vi "PIM Version.vi"() -> ()   [LabVIEW 2011]
uses:
  SI.LIB/OGAB Version.ctl
  server/database/Fields/Field Record.ctl
  server/database/Fields/Field DataTypes.ctl
  server/database/Fields/Field NextItem.ctl
panel:
  in  "Fields":T1[](array[typedef])=[{"ixField"=0, "iSequenceOrder"=0, "sxFieldId"="ALC", "sxSequenceId"="", "sDisplayName"="ALC", "sValue"="0", "sUnits"="", "nDataType"=enum."numeric", "nNextItem"=enum."Reset", "fSystem"=TRUE, "fSystemValue"=TRUE, "fRequired"=TRUE, "fSetAtTest"=TRUE, "fTestField"=TRUE, "fDeleted"=FALSE, "fIndexed"=FALSE, "fFreeList"=FALSE}, {"ixField"=0, "iSequenceOrder"=0, "sxFieldId"="Averaging", "sxSequenceId"="", "sDisplayName"="Averaging", "sValue"="None\tNone\tMinimum\tNormal\tHigh\tMaximum", "sUnits"="", "nDataType"=enum."list", "nNextItem"=enum."Reset", "fSystem"=TRUE, "fSystemValue"=TRUE, "fRequired"=TRUE, "fSetAtTest"=TRUE, "fTestField"=TRUE, "fDeleted"=FALSE, "fIndexed"=FALSE, "fFreeList"=FALSE}, {"ixField"=0, "iSequenceOrder"=0, "sxFieldId"="C1_Requested", "sxSequenceId"="", "sDisplayName"="C1 Requested", "sValue"="0", "sUnits"="dBm", "nDataType"=enum."numeric", "nNextItem"=enum."Reset", "fSystem"=TRUE, "fSystemValue"=TRUE, "fRequired"=TRUE, "fSetAtTest"=TRUE, "fTestField"=TRUE, "fDeleted"=FALSE, "fIndexed"=FALSE, "fFreeList"=FALSE}, {"ixField"=0, "iSequenceOrder"=0, "sxFieldId"="C2_Requested", "sxSequenceId"="", "sDisplayName"="C2 Requested", "sValue"="0", "sUnits"="dBm", "nDataType"=enum."numeric", "nNextItem"=enum."Reset", "fSystem"=TRUE, "fSystemValue"=TRUE, "fRequired"=TRUE, "fSetAtTest"=TRUE, "fTestField"=TRUE, "fDeleted"=FALSE, "fIndexed"=FALSE, "fFreeList"=FALSE}, {"ixField"=0, "iSequenceOrder"=0, "sxFieldId"="Calibration_Status", "sxSequenceId"="", "sDisplayName"="Calibration Status", "sValue"="0", "sUnits"="", "nDataType"=enum."numeric", "nNextItem"=enum."Reset", "fSystem"=TRUE, "fSystemValue"=TRUE, "fRequired"=TRUE, "fSetAtTest"=TRUE, "fTestField"=TRUE, "fDeleted"=FALSE, "fIndexed"=FALSE, "fFreeList"=FALSE}, {"ixField"=0, "iSequenceOrder"=0, "sxFieldId"="Cycles", "sxSequenceId"="", "sDisplayName"="Cycles", "sValue"="0", "sUnits"="", "nDataType"=enum."numeric", "nNextItem"=enum."Reset", "fSystem"=TRUE, "fSystemValue"=TRUE, "fRequired"=TRUE, "fSetAtTest"=TRUE, "fTestField"=TRUE, "fDeleted"=FALSE, "fIndexed"=FALSE, "fFreeList"=FALSE}, {"ixField"=0, "iSequenceOrder"=0, "sxFieldId"="DUT_Port", "sxSequenceId"="", "sDisplayName"="DUT Port", "sValue"="Port 1\tPort 1\tPort 2", "sUnits"="", "nDataType"=enum."list", "nNextItem"=enum."Reset", "fSystem"=TRUE, "fSystemValue"=TRUE, "fRequired"=TRUE, "fSetAtTest"=TRUE, "fTestField"=TRUE, "fDeleted"=FALSE, "fIndexed"=FALSE, "fFreeList"=FALSE}, {"ixField"=0, "iSequenceOrder"=0, "sxFieldId"="Display_Units_IM", "sxSequenceId"="", "sDisplayName"="Display Units IM", "sValue"="dBm\tdBm\tdBc", "sUnits"="", "nDataType"=enum."list", "nNextItem"=enum."Reset", "fSystem"=TRUE, "fSystemValue"=TRUE, "fRequired"=TRUE, "fSetAtTest"=TRUE, "fTestField"=TRUE, "fDeleted"=FALSE, "fIndexed"=FALSE, "fFreeList"=FALSE}, {"ixField"=0, "iSequenceOrder"=0, "sxFieldId"="Display_Units_Power", "sxSequenceId"="", "sDisplayName"="Display Units Power", "sValue"="dBm\tdBm\tWatts", "sUnits"="", "nDataType"=enum."list", "nNextItem"=enum."Reset", "fSystem"=TRUE, "fSystemValue"=TRUE, "fRequired"=TRUE, "fSetAtTest"=TRUE, "fTestField"=TRUE, "fDeleted"=FALSE, "fIndexed"=FALSE, "fFreeList"=FALSE}, {"ixField"=0, "iSequenceOrder"=0, "sxFieldId"="Display_Units_Samples", "sxSequenceId"="", "sDisplayName"="Display Units Samples", "sValue"="Sample(s)\tSample(s)\tSecond(s)\tSweep(s)", "sUnits"="", "nDataType"=enum."list", "nNextItem"=enum."Reset", "fSystem"=TRUE, "fSystemValue"=TRUE, "fRequired"=TRUE, "fSetAtTest"=TRUE, "fTestField"=TRUE, "fDeleted"=FALSE, "fIndexed"=FALSE, "fFreeList"=FALSE}, {"ixField"=0, "iSequenceOrder"=0, "sxFieldId"="IM11_Frequency_Average", "sxSequenceId"="", "sDisplayName"="IM11 Frequency Average", "sValue"="0", "sUnits"="MHz", "nDataType"=enum."numeric", "nNextItem"=enum."Reset", "fSystem"=TRUE, "fSystemValue"=TRUE, "fRequired"=TRUE, "fSetAtTest"=TRUE, "fTestField"=TRUE, "fDeleted"=FALSE, "fIndexed"=FALSE, "fFreeList"=FALSE}, {"ixField"=0, "iSequenceOrder"=0, "sxFieldId"="IM11_Frequency_Maximum", "sxSequenceId"="", "sDisplayName"="IM11 Frequency Maximum", "sValue"="0", "sUnits"="MHz", "nDataType"=enum."numeric", "nNextItem"=enum."Reset", "fSystem"=TRUE, "fSystemValue"=TRUE, "fRequired"=TRUE, "fSetAtTest"=TRUE, "fTestField"=TRUE, "fDeleted"=FALSE, "fIndexed"=FALSE, "fFreeList"=FALSE}, {"ixField"=0, "iSequenceOrder"=0, "sxFieldId"="IM11_Frequency_Minimum", "sxSequenceId"="", "sDisplayName"="IM11 Frequency Minimum", "sValue"="0", "sUnits"="MHz", "nDataType"=enum."numeric", "nNextItem"=enum."Reset", "fSystem"=TRUE, "fSystemValue"=TRUE, "fRequired"=TRUE, "fSetAtTest"=TRUE, "fTestField"=TRUE, "fDeleted"=FALSE, "fIndexed"=FALSE, "fFreeList"=FALSE}, {"ixField"=0, "iSequenceOrder"=0, "sxFieldId"="IM11_Frequency_Standard_Deviation", "sxSequenceId"="", "sDisplayName"="IM11 Frequency Standard Deviation", "sValue"="0", "sUnits"="MHz", "nDataType"=enum."numeric", "nNextItem"=enum."Reset", "fSystem"=TRUE, "fSystemValue"=TRUE, "fRequired"=TRUE, "fSetAtTest"=TRUE, "fTestField"=TRUE, "fDeleted"=FALSE, "fIndexed"=FALSE, "fFreeList"=FALSE}, {"ixField"=0, "iSequenceOrder"=0, "sxFieldId"="IM11_Power_1_Average", "sxSequenceId"="", "sDisplayName"="IM11 Power 1 Average", "sValue"="0", "sUnits"="dBm", "nDataType"=enum."numeric", "nNextItem"=enum."Reset", "fSystem"=TRUE, "fSystemValue"=TRUE, "fRequired"=TRUE, "fSetAtTest"=TRUE, "fTestField"=TRUE, "fDeleted"=FALSE, "fIndexed"=FALSE, "fFreeList"=FALSE}, {"ixField"=0, "iSequenceOrder"=0, "sxFieldId"="IM11_Power_1_Maximum", "sxSequenceId"="", "sDisplayName"="IM11 Power 1 Maximum", "sValue"="0", "sUnits"="dBm", "nDataType"=enum."numeric", "nNextItem"=enum."Reset", "fSystem"=TRUE, "fSystemValue"=TRUE, "fRequired"=TRUE, "fSetAtTest"=TRUE, "fTestField"=TRUE, "fDeleted"=FALSE, "fIndexed"=FALSE, "fFreeList"=FALSE}, {"ixField"=0, "iSequenceOrder"=0, "sxFieldId"="IM11_Power_1_Minimum", "sxSequenceId"="", "sDisplayName"="IM11 Power 1 Minimum", "sValue"="0", "sUnits"="dBm", "nDataType"=enum."numeric", "nNextItem"=enum."Reset", "fSystem"=TRUE, "fSystemValue"=TRUE, "fRequired"=TRUE, "fSetAtTest"=TRUE, "fTestField"=TRUE, "fDeleted"=FALSE, "fIndexed"=FALSE, "fFreeList"=FALSE}, {"ixField"=0, "iSequenceOrder"=0, "sxFieldId"="IM11_Power_1_Standard_Deviation", "sxSequenceId"="", "sDisplayName"="IM11 Power 1 Standard Deviation", "sValue"="0", "sUnits"="dBm", "nDataType"=enum."numeric", "nNextItem"=enum."Reset", "fSystem"=TRUE, "fSystemValue"=TRUE, "fRequired"=TRUE, "fSetAtTest"=TRUE, "fTestField"=TRUE, "fDeleted"=FALSE, "fIndexed"=FALSE, "fFreeList"=FALSE}, {"ixField"=0, "iSequenceOrder"=0, "sxFieldId"="IM11_Power_2_Average", "sxSequenceId"="", "sDisplayName"="IM11 Power 2 Average", "sValue"="0", "sUnits"="dBc", "nDataType"=enum."numeric", "nNextItem"=enum."Reset", "fSystem"=TRUE, "fSystemValue"=TRUE, "fRequired"=TRUE, "fSetAtTest"=TRUE, "fTestField"=TRUE, "fDeleted"=FALSE, "fIndexed"=FALSE, "fFreeList"=FALSE}, {"ixField"=0, "iSequenceOrder"=0, "sxFieldId"="IM11_Power_2_Maximum", "sxSequenceId"="", "sDisplayName"="IM11 Power 2 Maximum", "sValue"="0", "sUnits"="dBc", "nDataType"=enum."numeric", "nNextItem"=enum."Reset", "fSystem"=TRUE, "fSystemValue"=TRUE, "fRequired"=TRUE, "fSetAtTest"=TRUE, "fTestField"=TRUE, "fDeleted"=FALSE, "fIndexed"=FALSE, "fFreeList"=FALSE}, {"ixField"=0, "iSequenceOrder"=0, "sxFieldId"="IM11_Power_2_Minimum", "sxSequenceId"="", "sDisplayName"="IM11 Power 2 Minimum", "sValue"="0", "sUnits"="dBc", "nDataType"=enum."numeric", "nNextItem"=enum."Reset", "fSystem"=TRUE, "fSystemValue"=TRUE, "fRequired"=TRUE, "fSetAtTest"=TRUE, "fTestField"=TRUE, "fDeleted"=FALSE, "fIndexed"=FALSE, "fFreeList"=FALSE}, {"ixField"=0, "iSequenceOrder"=0, "sxFieldId"="IM11_Power_2_Standard_Deviation", "sxSequenceId"="", "sDisplayName"="IM11 Power 2 Standard Deviation", "sValue"="0", "sUnits"="dBc", "nDataType"=enum."numeric", "nNextItem"=enum."Reset", "fSystem"=TRUE, "fSystemValue"=TRUE, "fRequired"=TRUE, "fSetAtTest"=TRUE, "fTestField"=TRUE, "fDeleted"=FALSE, "fIndexed"=FALSE, "fFreeList"=FALSE}, {"ixField"=0, "iSequenceOrder"=0, "sxFieldId"="IM13_Frequency_Average", "sxSequenceId"="", "sDisplayName"="IM13 Frequency Average", "sValue"="0", "sUnits"="MHz", "nDataType"=enum."numeric", "nNextItem"=enum."Reset", "fSystem"=TRUE, "fSystemValue"=TRUE, "fRequired"=TRUE, "fSetAtTest"=TRUE, "fTestField"=TRUE, "fDeleted"=FALSE, "fIndexed"=FALSE, "fFreeList"=FALSE}, {"ixField"=0, "iSequenceOrder"=0, "sxFieldId"="IM13_Frequency_Maximum", "sxSequenceId"="", "sDisplayName"="IM13 Frequency Maximum", "sValue"="0", "sUnits"="MHz", "nDataType"=enum."numeric", "nNextItem"=enum."Reset", "fSystem"=TRUE, "fSystemValue"=TRUE, "fRequired"=TRUE, "fSetAtTest"=TRUE, "fTestField"=TRUE, "fDeleted"=FALSE, "fIndexed"=FALSE, "fFreeList"=FALSE}, {"ixField"=0, "iSequenceOrder"=0, "sxFieldId"="IM13_Frequency_Minimum", "sxSequenceId"="", "sDisplayName"="IM13 Frequency Minimum", "sValue"="0", "sUnits"="MHz", "nDataType"=enum."numeric", "nNextItem"=enum."Reset", "fSystem"=TRUE, "fSystemValue"=TRUE, "fRequired"=TRUE, "fSetAtTest"=TRUE, "fTestField"=TRUE, "fDeleted"=FALSE, "fIndexed"=FALSE, "fFreeList"=FALSE}, {"ixField"=0, "iSequenceOrder"=0, "sxFieldId"="IM13_Frequency_Standard_Deviation", "sxSequenceId"="", "sDisplayName"="IM13 Frequency Standard Deviation", "sValue"="0", "sUnits"="MHz", "nDataType"=enum."numeric", "nNextItem"=enum."Reset", "fSystem"=TRUE, "fSystemValue"=TRUE, "fRequired"=TRUE, "fSetAtTest"=TRUE, "fTestField"=TRUE, "fDeleted"=FALSE, "fIndexed"=FALSE, "fFreeList"=FALSE}, {"ixField"=0, "iSequenceOrder"=0, "sxFieldId"="IM13_Power_1_Average", "sxSequenceId"="", "sDisplayName"="IM13 Power 1 Average", "sValue"="0", "sUnits"="dBm", "nDataType"=enum."numeric", "nNextItem"=enum."Reset", "fSystem"=TRUE, "fSystemValue"=TRUE, "fRequired"=TRUE, "fSetAtTest"=TRUE, "fTestField"=TRUE, "fDeleted"=FALSE, "fIndexed"=FALSE, "fFreeList"=FALSE}, {"ixField"=0, "iSequenceOrder"=0, "sxFieldId"="IM13_Power_1_Maximum", "sxSequenceId"="", "sDisplayName"="IM13 Power 1 Maximum", "sValue"="0", "sUnits"="dBm", "nDataType"=enum."numeric", "nNextItem"=enum."Reset", "fSystem"=TRUE, "fSystemValue"=TRUE, "fRequired"=TRUE, "fSetAtTest"=TRUE, "fTestField"=TRUE, "fDeleted"=FALSE, "fIndexed"=FALSE, "fFreeList"=FALSE}, {"ixField"=0, "iSequenceOrder"=0, "sxFieldId"="IM13_Power_1_Minimum", "sxSequenceId"="", "sDisplayName"="IM13 Power 1 Minimum", "sValue"="0", "sUnits"="dBm", "nDataType"=enum."numeric", "nNextItem"=enum."Reset", "fSystem"=TRUE, "fSystemValue"=TRUE, "fRequired"=TRUE, "fSetAtTest"=TRUE, "fTestField"=TRUE, "fDeleted"=FALSE, "fIndexed"=FALSE, "fFreeList"=FALSE}, {"ixField"=0, "iSequenceOrder"=0, "sxFieldId"="IM13_Power_1_Standard_Deviation", "sxSequenceId"="", "sDisplayName"="IM13 Power 1 Standard Deviation", "sValue"="0", "sUnits"="dBm", "nDataType"=enum."numeric", "nNextItem"=enum."Reset", "fSystem"=TRUE, "fSystemValue"=TRUE, "fRequired"=TRUE, "fSetAtTest"=TRUE, "fTestField"=TRUE, "fDeleted"=FALSE, "fIndexed"=FALSE, "fFreeList"=FALSE}, {"ixField"=0, "iSequenceOrder"=0, "sxFieldId"="IM13_Power_2_Average", "sxSequenceId"="", "sDisplayName"="IM13 Power 2 Average", "sValue"="0", "sUnits"="dBc", "nDataType"=enum."numeric", "nNextItem"=enum."Reset", "fSystem"=TRUE, "fSystemValue"=TRUE, "fRequired"=TRUE, "fSetAtTest"=TRUE, "fTestField"=TRUE, "fDeleted"=FALSE, "fIndexed"=FALSE, "fFreeList"=FALSE}, {"ixField"=0, "iSequenceOrder"=0, "sxFieldId"="IM13_Power_2_Maximum", "sxSequenceId"="", "sDisplayName"="IM13 Power 2 Maximum", "sValue"="0", "sUnits"="dBc", "nDataType"=enum."numeric", "nNextItem"=enum."Reset", "fSystem"=TRUE, "fSystemValue"=TRUE, "fRequired"=TRUE, "fSetAtTest"=TRUE, "fTestField"=TRUE, "fDeleted"=FALSE, "fIndexed"=FALSE, "fFreeList"=FALSE}, {"ixField"=0, "iSequenceOrder"=0, "sxFieldId"="IM13_Power_2_Minimum", "sxSequenceId"="", "sDisplayName"="IM13 Power 2 Minimum", "sValue"="0", "sUnits"="dBc", "nDataType"=enum."numeric", "nNextItem"=enum."Reset", "fSystem"=TRUE, "fSystemValue"=TRUE, "fRequired"=TRUE, "fSetAtTest"=TRUE, "fTestField"=TRUE, "fDeleted"=FALSE, "fIndexed"=FALSE, "fFreeList"=FALSE}, {"ixField"=0, "iSequenceOrder"=0, "sxFieldId"="IM13_Power_2_Standard_Deviation", "sxSequenceId"="", "sDisplayName"="IM13 Power 2 Standard Deviation", "sValue"="0", "sUnits"="dBc", "nDataType"=enum."numeric", "nNextItem"=enum."Reset", "fSystem"=TRUE, "fSystemValue"=TRUE, "fRequired"=TRUE, "fSetAtTest"=TRUE, "fTestField"=TRUE, "fDeleted"=FALSE, "fIndexed"=FALSE, "fFreeList"=FALSE}, {"ixField"=0, "iSequenceOrder"=0, "sxFieldId"="IM15_Frequency_Average", "sxSequenceId"="", "sDisplayName"="IM15 Frequency Average", "sValue"="0", "sUnits"="MHz", "nDataType"=enum."numeric", "nNextItem"=enum."Reset", "fSystem"=TRUE, "fSystemValue"=TRUE, "fRequired"=TRUE, "fSetAtTest"=TRUE, "fTestField"=TRUE, "fDeleted"=FALSE, "fIndexed"=FALSE, "fFreeList"=FALSE}, {"ixField"=0, "iSequenceOrder"=0, "sxFieldId"="IM15_Frequency_Maximum", "sxSequenceId"="", "sDisplayName"="IM15 Frequency Maximum", "sValue"="0", "sUnits"="MHz", "nDataType"=enum."numeric", "nNextItem"=enum."Reset", "fSystem"=TRUE, "fSystemValue"=TRUE, "fRequired"=TRUE, "fSetAtTest"=TRUE, "fTestField"=TRUE, "fDeleted"=FALSE, "fIndexed"=FALSE, "fFreeList"=FALSE}, {"ixField"=0, "iSequenceOrder"=0, "sxFieldId"="IM15_Frequency_Minimum", "sxSequenceId"="", "sDisplayName"="IM15 Frequency Minimum", "sValue"="0", "sUnits"="MHz", "nDataType"=enum."numeric", "nNextItem"=enum."Reset", "fSystem"=TRUE, "fSystemValue"=TRUE, "fRequired"=TRUE, "fSetAtTest"=TRUE, "fTestField"=TRUE, "fDeleted"=FALSE, "fIndexed"=FALSE, "fFreeList"=FALSE}, {"ixField"=0, "iSequenceOrder"=0, "sxFieldId"="IM15_Frequency_Standard_Deviation", "sxSequenceId"="", "sDisplayName"="IM15 Frequency Standard Deviation", "sValue"="0", "sUnits"="MHz", "nDataType"=enum."numeric", "nNextItem"=enum."Reset", "fSystem"=TRUE, "fSystemValue"=TRUE, "fRequired"=TRUE, "fSetAtTest"=TRUE, "fTestField"=TRUE, "fDeleted"=FALSE, "fIndexed"=FALSE, "fFreeList"=FALSE}, {"ixField"=0, "iSequenceOrder"=0, "sxFieldId"="IM15_Power_1_Average", "sxSequenceId"="", "sDisplayName"="IM15 Power 1 Average", "sValue"="0", "sUnits"="dBm", "nDataType"=enum."numeric", "nNextItem"=enum."Reset", "fSystem"=TRUE, "fSystemValue"=TRUE, "fRequired"=TRUE, "fSetAtTest"=TRUE, "fTestField"=TRUE, "fDeleted"=FALSE, "fIndexed"=FALSE, "fFreeList"=FALSE}, {"ixField"=0, "iSequenceOrder"=0, "sxFieldId"="IM15_Power_1_Maximum", "sxSequenceId"="", "sDisplayName"="IM15 Power 1 Maximum", "sValue"="0", "sUnits"="dBm", "nDataType"=enum."numeric", "nNextItem"=enum."Reset", "fSystem"=TRUE, "fSystemValue"=TRUE, "fRequired"=TRUE, "fSetAtTest"=TRUE, "fTestField"=TRUE, "fDeleted"=FALSE, "fIndexed"=FALSE, "fFreeList"=FALSE}, {"ixField"=0, "iSequenceOrder"=0, "sxFieldId"="IM15_Power_1_Minimum", "sxSequenceId"="", "sDisplayName"="IM15 Power 1 Minimum", "sValue"="0", "sUnits"="dBm", "nDataType"=enum."numeric", "nNextItem"=enum."Reset", "fSystem"=TRUE, "fSystemValue"=TRUE, "fRequired"=TRUE, "fSetAtTest"=TRUE, "fTestField"=TRUE, "fDeleted"=FALSE, "fIndexed"=FALSE, "fFreeList"=FALSE}, {"ixField"=0, "iSequenceOrder"=0, "sxFieldId"="IM15_Power_1_Standard_Deviation", "sxSequenceId"="", "sDisplayName"="IM15 Power 1 Standard Deviation", "sValue"="0", "sUnits"="dBm", "nDataType"=enum."numeric", "nNextItem"=enum."Reset", "fSystem"=TRUE, "fSystemValue"=TRUE, "fRequired"=TRUE, "fSetAtTest"=TRUE, "fTestField"=TRUE, "fDeleted"=FALSE, "fIndexed"=FALSE, "fFreeList"=FALSE}, {"ixField"=0, "iSequenceOrder"=0, "sxFieldId"="IM15_Power_2_Average", "sxSequenceId"="", "sDisplayName"="IM15 Power 2 Average", "sValue"="0", "sUnits"="dBc", "nDataType"=enum."numeric", "nNextItem"=enum."Reset", "fSystem"=TRUE, "fSystemValue"=TRUE, "fRequired"=TRUE, "fSetAtTest"=TRUE, "fTestField"=TRUE, "fDeleted"=FALSE, "fIndexed"=FALSE, "fFreeList"=FALSE}, {"ixField"=0, "iSequenceOrder"=0, "sxFieldId"="IM15_Power_2_Maximum", "sxSequenceId"="", "sDisplayName"="IM15 Power 2 Maximum", "sValue"="0", "sUnits"="dBc", "nDataType"=enum."numeric", "nNextItem"=enum."Reset", "fSystem"=TRUE, "fSystemValue"=TRUE, "fRequired"=TRUE, "fSetAtTest"=TRUE, "fTestField"=TRUE, "fDeleted"=FALSE, "fIndexed"=FALSE, "fFreeList"=FALSE}, {"ixField"=0, "iSequenceOrder"=0, "sxFieldId"="IM15_Power_2_Minimum", "sxSequenceId"="", "sDisplayName"="IM15 Power 2 Minimum", "sValue"="0", "sUnits"="dBc", "nDataType"=enum."numeric", "nNextItem"=enum."Reset", "fSystem"=TRUE, "fSystemValue"=TRUE, "fRequired"=TRUE, "fSetAtTest"=TRUE, "fTestField"=TRUE, "fDeleted"=FALSE, "fIndexed"=FALSE, "fFreeList"=FALSE}, {"ixField"=0, "iSequenceOrder"=0, "sxFieldId"="IM15_Power_2_Standard_Deviation", "sxSequenceId"="", "sDisplayName"="IM15 Power 2 Standard Deviation", "sValue"="0", "sUnits"="dBc", "nDataType"=enum."numeric", "nNextItem"=enum."Reset", "fSystem"=TRUE, "fSystemValue"=TRUE, "fRequired"=TRUE, "fSetAtTest"=TRUE, "fTestField"=TRUE, "fDeleted"=FALSE, "fIndexed"=FALSE, "fFreeList"=FALSE}, {"ixField"=0, "iSequenceOrder"=0, "sxFieldId"="IM17_Frequency_Average", "sxSequenceId"="", "sDisplayName"="IM17 Frequency Average", "sValue"="0", "sUnits"="MHz", "nDataType"=enum."numeric", "nNextItem"=enum."Reset", "fSystem"=TRUE, "fSystemValue"=TRUE, "fRequired"=TRUE, "fSetAtTest"=TRUE, "fTestField"=TRUE, "fDeleted"=FALSE, "fIndexed"=FALSE, "fFreeList"=FALSE}, {"ixField"=0, "iSequenceOrder"=0, "sxFieldId"="IM17_Frequency_Maximum", "sxSequenceId"="", "sDisplayName"="IM17 Frequency Maximum", "sValue"="0", "sUnits"="MHz", "nDataType"=enum."numeric", "nNextItem"=enum."Reset", "fSystem"=TRUE, "fSystemValue"=TRUE, "fRequired"=TRUE, "fSetAtTest"=TRUE, "fTestField"=TRUE, "fDeleted"=FALSE, "fIndexed"=FALSE, "fFreeList"=FALSE}, {"ixField"=0, "iSequenceOrder"=0, "sxFieldId"="IM17_Frequency_Minimum", "sxSequenceId"="", "sDisplayName"="IM17 Frequency Minimum", "sValue"="0", "sUnits"="MHz", "nDataType"=enum."numeric", "nNextItem"=enum."Reset", "fSystem"=TRUE, "fSystemValue"=TRUE, "fRequired"=TRUE, "fSetAtTest"=TRUE, "fTestField"=TRUE, "fDeleted"=FALSE, "fIndexed"=FALSE, "fFreeList"=FALSE}, {"ixField"=0, "iSequenceOrder"=0, "sxFieldId"="IM17_Frequency_Standard_Deviation", "sxSequenceId"="", "sDisplayName"="IM17 Frequency Standard Deviation", "sValue"="0", "sUnits"="MHz", "nDataType"=enum."numeric", "nNextItem"=enum."Reset", "fSystem"=TRUE, "fSystemValue"=TRUE, "fRequired"=TRUE, "fSetAtTest"=TRUE, "fTestField"=TRUE, "fDeleted"=FALSE, "fIndexed"=FALSE, "fFreeList"=FALSE}, {"ixField"=0, "iSequenceOrder"=0, "sxFieldId"="IM17_Power_1_Average", "sxSequenceId"="", "sDisplayName"="IM17 Power 1 Average", "sValue"="0", "sUnits"="dBm", "nDataType"=enum."numeric", "nNextItem"=enum."Reset", "fSystem"=TRUE, "fSystemValue"=TRUE, "fRequired"=TRUE, "fSetAtTest"=TRUE, "fTestField"=TRUE, "fDeleted"=FALSE, "fIndexed"=FALSE, "fFreeList"=FALSE}, {"ixField"=0, "iSequenceOrder"=0, "sxFieldId"="IM17_Power_1_Maximum", "sxSequenceId"="", "sDisplayName"="IM17 Power 1 Maximum", "sValue"="0", "sUnits"="dBm", "nDataType"=enum."numeric", "nNextItem"=enum."Reset", "fSystem"=TRUE, "fSystemValue"=TRUE, "fRequired"=TRUE, "fSetAtTest"=TRUE, "fTestField"=TRUE, "fDeleted"=FALSE, "fIndexed"=FALSE, "fFreeList"=FALSE}, {"ixField"=0, "iSequenceOrder"=0, "sxFieldId"="IM17_Power_1_Minimum", "sxSequenceId"="", "sDisplayName"="IM17 Power 1 Minimum", "sValue"="0", "sUnits"="dBm", "nDataType"=enum."numeric", "nNextItem"=enum."Reset", "fSystem"=TRUE, "fSystemValue"=TRUE, "fRequired"=TRUE, "fSetAtTest"=TRUE, "fTestField"=TRUE, "fDeleted"=FALSE, "fIndexed"=FALSE, "fFreeList"=FALSE}, {"ixField"=0, "iSequenceOrder"=0, "sxFieldId"="IM17_Power_1_Standard_Deviation", "sxSequenceId"="", "sDisplayName"="IM17 Power 1 Standard Deviation", "sValue"="0", "sUnits"="dBm", "nDataType"=enum."numeric", "nNextItem"=enum."Reset", "fSystem"=TRUE, "fSystemValue"=TRUE, "fRequired"=TRUE, "fSetAtTest"=TRUE, "fTestField"=TRUE, "fDeleted"=FALSE, "fIndexed"=FALSE, "fFreeList"=FALSE}, {"ixField"=0, "iSequenceOrder"=0, "sxFieldId"="IM17_Power_2_Average", "sxSequenceId"="", "sDisplayName"="IM17 Power 2 Average", "sValue"="0", "sUnits"="dBc", "nDataType"=enum."numeric", "nNextItem"=enum."Reset", "fSystem"=TRUE, "fSystemValue"=TRUE, "fRequired"=TRUE, "fSetAtTest"=TRUE, "fTestField"=TRUE, "fDeleted"=FALSE, "fIndexed"=FALSE, "fFreeList"=FALSE}, {"ixField"=0, "iSequenceOrder"=0, "sxFieldId"="IM17_Power_2_Maximum", "sxSequenceId"="", "sDisplayName"="IM17 Power 2 Maximum", "sValue"="0", "sUnits"="dBc", "nDataType"=enum."numeric", "nNextItem"=enum."Reset", "fSystem"=TRUE, "fSystemValue"=TRUE, "fRequired"=TRUE, "fSetAtTest"=TRUE, "fTestField"=TRUE, "fDeleted"=FALSE, "fIndexed"=FALSE, "fFreeList"=FALSE}, {"ixField"=0, "iSequenceOrder"=0, "sxFieldId"="IM17_Power_2_Minimum", "sxSequenceId"="", "sDisplayName"="IM17 Power 2 Minimum", "sValue"="0", "sUnits"="dBc", "nDataType"=enum."numeric", "nNextItem"=enum."Reset", "fSystem"=TRUE, "fSystemValue"=TRUE, "fRequired"=TRUE, "fSetAtTest"=TRUE, "fTestField"=TRUE, "fDeleted"=FALSE, "fIndexed"=FALSE, "fFreeList"=FALSE}, {"ixField"=0, "iSequenceOrder"=0, "sxFieldId"="IM17_Power_2_Standard_Deviation", "sxSequenceId"="", "sDisplayName"="IM17 Power 2 Standard Deviation", "sValue"="0", "sUnits"="dBc", "nDataType"=enum."numeric", "nNextItem"=enum."Reset", "fSystem"=TRUE, "fSystemValue"=TRUE, "fRequired"=TRUE, "fSetAtTest"=TRUE, "fTestField"=TRUE, "fDeleted"=FALSE, "fIndexed"=FALSE, "fFreeList"=FALSE}, {"ixField"=0, "iSequenceOrder"=0, "sxFieldId"="IM19_Frequency_Average", "sxSequenceId"="", "sDisplayName"="IM19 Frequency Average", "sValue"="0", "sUnits"="MHz", "nDataType"=enum."numeric", "nNextItem"=enum."Reset", "fSystem"=TRUE, "fSystemValue"=TRUE, "fRequired"=TRUE, "fSetAtTest"=TRUE, "fTestField"=TRUE, "fDeleted"=FALSE, "fIndexed"=FALSE, "fFreeList"=FALSE}, {"ixField"=0, "iSequenceOrder"=0, "sxFieldId"="IM19_Frequency_Maximum", "sxSequenceId"="", "sDisplayName"="IM19 Frequency Maximum", "sValue"="0", "sUnits"="MHz", "nDataType"=enum."numeric", "nNextItem"=enum."Reset", "fSystem"=TRUE, "fSystemValue"=TRUE, "fRequired"=TRUE, "fSetAtTest"=TRUE, "fTestField"=TRUE, "fDeleted"=FALSE, "fIndexed"=FALSE, "fFreeList"=FALSE}, {"ixField"=0, "iSequenceOrder"=0, "sxFieldId"="IM19_Frequency_Minimum", "sxSequenceId"="", "sDisplayName"="IM19 Frequency Minimum", "sValue"="0", "sUnits"="MHz", "nDataType"=enum."numeric", "nNextItem"=enum."Reset", "fSystem"=TRUE, "fSystemValue"=TRUE, "fRequired"=TRUE, "fSetAtTest"=TRUE, "fTestField"=TRUE, "fDeleted"=FALSE, "fIndexed"=FALSE, "fFreeList"=FALSE}, {"ixField"=0, "iSequenceOrder"=0, "sxFieldId"="IM19_Frequency_Standard_Deviation", "sxSequenceId"="", "sDisplayName"="IM19 Frequency Standard Deviation", "sValue"="0", "sUnits"="MHz", "nDataType"=enum."numeric", "nNextItem"=enum."Reset", "fSystem"=TRUE, "fSystemValue"=TRUE, "fRequired"=TRUE, "fSetAtTest"=TRUE, "fTestField"=TRUE, "fDeleted"=FALSE, "fIndexed"=FALSE, "fFreeList"=FALSE}, {"ixField"=0, "iSequenceOrder"=0, "sxFieldId"="IM19_Power_1_Average", "sxSequenceId"="", "sDisplayName"="IM19 Power 1 Average", "sValue"="0", "sUnits"="dBm", "nDataType"=enum."numeric", "nNextItem"=enum."Reset", "fSystem"=TRUE, "fSystemValue"=TRUE, "fRequired"=TRUE, "fSetAtTest"=TRUE, "fTestField"=TRUE, "fDeleted"=FALSE, "fIndexed"=FALSE, "fFreeList"=FALSE}, {"ixField"=0, "iSequenceOrder"=0, "sxFieldId"="IM19_Power_1_Maximum", "sxSequenceId"="", "sDisplayName"="IM19 Power 1 Maximum", "sValue"="0", "sUnits"="dBm", "nDataType"=enum."numeric", "nNextItem"=enum."Reset", "fSystem"=TRUE, "fSystemValue"=TRUE, "fRequired"=TRUE, "fSetAtTest"=TRUE, "fTestField"=TRUE, "fDeleted"=FALSE, "fIndexed"=FALSE, "fFreeList"=FALSE}, {"ixField"=0, "iSequenceOrder"=0, "sxFieldId"="IM19_Power_1_Minimum", "sxSequenceId"="", "sDisplayName"="IM19 Power 1 Minimum", "sValue"="0", "sUnits"="dBm", "nDataType"=enum."numeric", "nNextItem"=enum."Reset", "fSystem"=TRUE, "fSystemValue"=TRUE, "fRequired"=TRUE, "fSetAtTest"=TRUE, "fTestField"=TRUE, "fDeleted"=FALSE, "fIndexed"=FALSE, "fFreeList"=FALSE}, {"ixField"=0, "iSequenceOrder"=0, "sxFieldId"="IM19_Power_1_Standard_Deviation", "sxSequenceId"="", "sDisplayName"="IM19 Power 1 Standard Deviation", "sValue"="0", "sUnits"="dBm", "nDataType"=enum."numeric", "nNextItem"=enum."Reset", "fSystem"=TRUE, "fSystemValue"=TRUE, "fRequired"=TRUE, "fSetAtTest"=TRUE, "fTestField"=TRUE, "fDeleted"=FALSE, "fIndexed"=FALSE, "fFreeList"=FALSE}, {"ixField"=0, "iSequenceOrder"=0, "sxFieldId"="IM19_Power_2_Average", "sxSequenceId"="", "sDisplayName"="IM19 Power 2 Average", "sValue"="0", "sUnits"="dBc", "nDataType"=enum."numeric", "nNextItem"=enum."Reset", "fSystem"=TRUE, "fSystemValue"=TRUE, "fRequired"=TRUE, "fSetAtTest"=TRUE, "fTestField"=TRUE, "fDeleted"=FALSE, "fIndexed"=FALSE, "fFreeList"=FALSE}, {"ixField"=0, "iSequenceOrder"=0, "sxFieldId"="IM19_Power_2_Maximum", "sxSequenceId"="", "sDisplayName"="IM19 Power 2 Maximum", "sValue"="0", "sUnits"="dBc", "nDataType"=enum."numeric", "nNextItem"=enum."Reset", "fSystem"=TRUE, "fSystemValue"=TRUE, "fRequired"=TRUE, "fSetAtTest"=TRUE, "fTestField"=TRUE, "fDeleted"=FALSE, "fIndexed"=FALSE, "fFreeList"=FALSE}, {"ixField"=0, "iSequenceOrder"=0, "sxFieldId"="IM19_Power_2_Minimum", "sxSequenceId"="", "sDisplayName"="IM19 Power 2 Minimum", "sValue"="0", "sUnits"="dBc", "nDataType"=enum."numeric", "nNextItem"=enum."Reset", "fSystem"=TRUE, "fSystemValue"=TRUE, "fRequired"=TRUE, "fSetAtTest"=TRUE, "fTestField"=TRUE, "fDeleted"=FALSE, "fIndexed"=FALSE, "fFreeList"=FALSE}, {"ixField"=0, "iSequenceOrder"=0, "sxFieldId"="IM19_Power_2_Standard_Deviation", "sxSequenceId"="", "sDisplayName"="IM19 Power 2 Standard Deviation", "sValue"="0", "sUnits"="dBc", "nDataType"=enum."numeric", "nNextItem"=enum."Reset", "fSystem"=TRUE, "fSystemValue"=TRUE, "fRequired"=TRUE, "fSetAtTest"=TRUE, "fTestField"=TRUE, "fDeleted"=FALSE, "fIndexed"=FALSE, "fFreeList"=FALSE}, {"ixField"=0, "iSequenceOrder"=0, "sxFieldId"="IM21_Frequency_Average", "sxSequenceId"="", "sDisplayName"="IM21 Frequency Average", "sValue"="0", "sUnits"="MHz", "nDataType"=enum."numeric", "nNextItem"=enum."Reset", "fSystem"=TRUE, "fSystemValue"=TRUE, "fRequired"=TRUE, "fSetAtTest"=TRUE, "fTestField"=TRUE, "fDeleted"=FALSE, "fIndexed"=FALSE, "fFreeList"=FALSE}, {"ixField"=0, "iSequenceOrder"=0, "sxFieldId"="IM21_Frequency_Maximum", "sxSequenceId"="", "sDisplayName"="IM21 Frequency Maximum", "sValue"="0", "sUnits"="MHz", "nDataType"=enum."numeric", "nNextItem"=enum."Reset", "fSystem"=TRUE, "fSystemValue"=TRUE, "fRequired"=TRUE, "fSetAtTest"=TRUE, "fTestField"=TRUE, "fDeleted"=FALSE, "fIndexed"=FALSE, "fFreeList"=FALSE}, {"ixField"=0, "iSequenceOrder"=0, "sxFieldId"="IM21_Frequency_Minimum", "sxSequenceId"="", "sDisplayName"="IM21 Frequency Minimum", "sValue"="0", "sUnits"="MHz", "nDataType"=enum."numeric", "nNextItem"=enum."Reset", "fSystem"=TRUE, "fSystemValue"=TRUE, "fRequired"=TRUE, "fSetAtTest"=TRUE, "fTestField"=TRUE, "fDeleted"=FALSE, "fIndexed"=FALSE, "fFreeList"=FALSE}, {"ixField"=0, "iSequenceOrder"=0, "sxFieldId"="IM21_Frequency_Standard_Deviation", "sxSequenceId"="", "sDisplayName"="IM21 Frequency Standard Deviation", "sValue"="0", "sUnits"="MHz", "nDataType"=enum."numeric", "nNextItem"=enum."Reset", "fSystem"=TRUE, "fSystemValue"=TRUE, "fRequired"=TRUE, "fSetAtTest"=TRUE, "fTestField"=TRUE, "fDeleted"=FALSE, "fIndexed"=FALSE, "fFreeList"=FALSE}, {"ixField"=0, "iSequenceOrder"=0, "sxFieldId"="IM21_Power_1_Average", "sxSequenceId"="", "sDisplayName"="IM21 Power 1 Average", "sValue"="0", "sUnits"="dBm", "nDataType"=enum."numeric", "nNextItem"=enum."Reset", "fSystem"=TRUE, "fSystemValue"=TRUE, "fRequired"=TRUE, "fSetAtTest"=TRUE, "fTestField"=TRUE, "fDeleted"=FALSE, "fIndexed"=FALSE, "fFreeList"=FALSE}, {"ixField"=0, "iSequenceOrder"=0, "sxFieldId"="IM21_Power_1_Maximum", "sxSequenceId"="", "sDisplayName"="IM21 Power 1 Maximum", "sValue"="0", "sUnits"="dBm", "nDataType"=enum."numeric", "nNextItem"=enum."Reset", "fSystem"=TRUE, "fSystemValue"=TRUE, "fRequired"=TRUE, "fSetAtTest"=TRUE, "fTestField"=TRUE, "fDeleted"=FALSE, "fIndexed"=FALSE, "fFreeList"=FALSE}, {"ixField"=0, "iSequenceOrder"=0, "sxFieldId"="IM21_Power_1_Minimum", "sxSequenceId"="", "sDisplayName"="IM21 Power 1 Minimum", "sValue"="0", "sUnits"="dBm", "nDataType"=enum."numeric", "nNextItem"=enum."Reset", "fSystem"=TRUE, "fSystemValue"=TRUE, "fRequired"=TRUE, "fSetAtTest"=TRUE, "fTestField"=TRUE, "fDeleted"=FALSE, "fIndexed"=FALSE, "fFreeList"=FALSE}, {"ixField"=0, "iSequenceOrder"=0, "sxFieldId"="IM21_Power_1_Standard_Deviation", "sxSequenceId"="", "sDisplayName"="IM21 Power 1 Standard Deviation", "sValue"="0", "sUnits"="dBm", "nDataType"=enum."numeric", "nNextItem"=enum."Reset", "fSystem"=TRUE, "fSystemValue"=TRUE, "fRequired"=TRUE, "fSetAtTest"=TRUE, "fTestField"=TRUE, "fDeleted"=FALSE, "fIndexed"=FALSE, "fFreeList"=FALSE}, {"ixField"=0, "iSequenceOrder"=0, "sxFieldId"="IM21_Power_2_Average", "sxSequenceId"="", "sDisplayName"="IM21 Power 2 Average", "sValue"="0", "sUnits"="dBc", "nDataType"=enum."numeric", "nNextItem"=enum."Reset", "fSystem"=TRUE, "fSystemValue"=TRUE, "fRequired"=TRUE, "fSetAtTest"=TRUE, "fTestField"=TRUE, "fDeleted"=FALSE, "fIndexed"=FALSE, "fFreeList"=FALSE}, {"ixField"=0, "iSequenceOrder"=0, "sxFieldId"="IM21_Power_2_Maximum", "sxSequenceId"="", "sDisplayName"="IM21 Power 2 Maximum", "sValue"="0", "sUnits"="dBc", "nDataType"=enum."numeric", "nNextItem"=enum."Reset", "fSystem"=TRUE, "fSystemValue"=TRUE, "fRequired"=TRUE, "fSetAtTest"=TRUE, "fTestField"=TRUE, "fDeleted"=FALSE, "fIndexed"=FALSE, "fFreeList"=FALSE}, {"ixField"=0, "iSequenceOrder"=0, "sxFieldId"="IM21_Power_2_Minimum", "sxSequenceId"="", "sDisplayName"="IM21 Power 2 Minimum", "sValue"="0", "sUnits"="dBc", "nDataType"=enum."numeric", "nNextItem"=enum."Reset", "fSystem"=TRUE, "fSystemValue"=TRUE, "fRequired"=TRUE, "fSetAtTest"=TRUE, "fTestField"=TRUE, "fDeleted"=FALSE, "fIndexed"=FALSE, "fFreeList"=FALSE}, {"ixField"=0, "iSequenceOrder"=0, "sxFieldId"="IM21_Power_2_Standard_Deviation", "sxSequenceId"="", "sDisplayName"="IM21 Power 2 Standard Deviation", "sValue"="0", "sUnits"="dBc", "nDataType"=enum."numeric", "nNextItem"=enum."Reset", "fSystem"=TRUE, "fSystemValue"=TRUE, "fRequired"=TRUE, "fSetAtTest"=TRUE, "fTestField"=TRUE, "fDeleted"=FALSE, "fIndexed"=FALSE, "fFreeList"=FALSE}, {"ixField"=0, "iSequenceOrder"=0, "sxFieldId"="IM23_Frequency_Average", "sxSequenceId"="", "sDisplayName"="IM23 Frequency Average", "sValue"="0", "sUnits"="MHz", "nDataType"=enum."numeric", "nNextItem"=enum."Reset", "fSystem"=TRUE, "fSystemValue"=TRUE, "fRequired"=TRUE, "fSetAtTest"=TRUE, "fTestField"=TRUE, "fDeleted"=FALSE, "fIndexed"=FALSE, "fFreeList"=FALSE}, {"ixField"=0, "iSequenceOrder"=0, "sxFieldId"="IM23_Frequency_Maximum", "sxSequenceId"="", "sDisplayName"="IM23 Frequency Maximum", "sValue"="0", "sUnits"="MHz", "nDataType"=enum."numeric", "nNextItem"=enum."Reset", "fSystem"=TRUE, "fSystemValue"=TRUE, "fRequired"=TRUE, "fSetAtTest"=TRUE, "fTestField"=TRUE, "fDeleted"=FALSE, "fIndexed"=FALSE, "fFreeList"=FALSE}, {"ixField"=0, "iSequenceOrder"=0, "sxFieldId"="IM23_Frequency_Minimum", "sxSequenceId"="", "sDisplayName"="IM23 Frequency Minimum", "sValue"="0", "sUnits"="MHz", "nDataType"=enum."numeric", "nNextItem"=enum."Reset", "fSystem"=TRUE, "fSystemValue"=TRUE, "fRequired"=TRUE, "fSetAtTest"=TRUE, "fTestField"=TRUE, "fDeleted"=FALSE, "fIndexed"=FALSE, "fFreeList"=FALSE}, {"ixField"=0, "iSequenceOrder"=0, "sxFieldId"="IM23_Frequency_Standard_Deviation", "sxSequenceId"="", "sDisplayName"="IM23 Frequency Standard Deviation", "sValue"="0", "sUnits"="MHz", "nDataType"=enum."numeric", "nNextItem"=enum."Reset", "fSystem"=TRUE, "fSystemValue"=TRUE, "fRequired"=TRUE, "fSetAtTest"=TRUE, "fTestField"=TRUE, "fDeleted"=FALSE, "fIndexed"=FALSE, "fFreeList"=FALSE}, {"ixField"=0, "iSequenceOrder"=0, "sxFieldId"="IM23_Power_1_Average", "sxSequenceId"="", "sDisplayName"="IM23 Power 1 Average", "sValue"="0", "sUnits"="dBm", "nDataType"=enum."numeric", "nNextItem"=enum."Reset", "fSystem"=TRUE, "fSystemValue"=TRUE, "fRequired"=TRUE, "fSetAtTest"=TRUE, "fTestField"=TRUE, "fDeleted"=FALSE, "fIndexed"=FALSE, "fFreeList"=FALSE}, {"ixField"=0, "iSequenceOrder"=0, "sxFieldId"="IM23_Power_1_Maximum", "sxSequenceId"="", "sDisplayName"="IM23 Power 1 Maximum", "sValue"="0", "sUnits"="dBm", "nDataType"=enum."numeric", "nNextItem"=enum."Reset", "fSystem"=TRUE, "fSystemValue"=TRUE, "fRequired"=TRUE, "fSetAtTest"=TRUE, "fTestField"=TRUE, "fDeleted"=FALSE, "fIndexed"=FALSE, "fFreeList"=FALSE}, {"ixField"=0, "iSequenceOrder"=0, "sxFieldId"="IM23_Power_1_Minimum", "sxSequenceId"="", "sDisplayName"="IM23 Power 1 Minimum", "sValue"="0", "sUnits"="dBm", "nDataType"=enum."numeric", "nNextItem"=enum."Reset", "fSystem"=TRUE, "fSystemValue"=TRUE, "fRequired"=TRUE, "fSetAtTest"=TRUE, "fTestField"=TRUE, "fDeleted"=FALSE, "fIndexed"=FALSE, "fFreeList"=FALSE}, {"ixField"=0, "iSequenceOrder"=0, "sxFieldId"="IM23_Power_1_Standard_Deviation", "sxSequenceId"="", "sDisplayName"="IM23 Power 1 Standard Deviation", "sValue"="0", "sUnits"="dBm", "nDataType"=enum."numeric", "nNextItem"=enum."Reset", "fSystem"=TRUE, "fSystemValue"=TRUE, "fRequired"=TRUE, "fSetAtTest"=TRUE, "fTestField"=TRUE, "fDeleted"=FALSE, "fIndexed"=FALSE, "fFreeList"=FALSE}, {"ixField"=0, "iSequenceOrder"=0, "sxFieldId"="IM23_Power_2_Average", "sxSequenceId"="", "sDisplayName"="IM23 Power 2 Average", "sValue"="0", "sUnits"="dBc", "nDataType"=enum."numeric", "nNextItem"=enum."Reset", "fSystem"=TRUE, "fSystemValue"=TRUE, "fRequired"=TRUE, "fSetAtTest"=TRUE, "fTestField"=TRUE, "fDeleted"=FALSE, "fIndexed"=FALSE, "fFreeList"=FALSE}, {"ixField"=0, "iSequenceOrder"=0, "sxFieldId"="IM23_Power_2_Maximum", "sxSequenceId"="", "sDisplayName"="IM23 Power 2 Maximum", "sValue"="0", "sUnits"="dBc", "nDataType"=enum."numeric", "nNextItem"=enum."Reset", "fSystem"=TRUE, "fSystemValue"=TRUE, "fRequired"=TRUE, "fSetAtTest"=TRUE, "fTestField"=TRUE, "fDeleted"=FALSE, "fIndexed"=FALSE, "fFreeList"=FALSE}, {"ixField"=0, "iSequenceOrder"=0, "sxFieldId"="IM23_Power_2_Minimum", "sxSequenceId"="", "sDisplayName"="IM23 Power 2 Minimum", "sValue"="0", "sUnits"="dBc", "nDataType"=enum."numeric", "nNextItem"=enum."Reset", "fSystem"=TRUE, "fSystemValue"=TRUE, "fRequired"=TRUE, "fSetAtTest"=TRUE, "fTestField"=TRUE, "fDeleted"=FALSE, "fIndexed"=FALSE, "fFreeList"=FALSE}, {"ixField"=0, "iSequenceOrder"=0, "sxFieldId"="IM23_Power_2_Standard_Deviation", "sxSequenceId"="", "sDisplayName"="IM23 Power 2 Standard Deviation", "sValue"="0", "sUnits"="dBc", "nDataType"=enum."numeric", "nNextItem"=enum."Reset", "fSystem"=TRUE, "fSystemValue"=TRUE, "fRequired"=TRUE, "fSetAtTest"=TRUE, "fTestField"=TRUE, "fDeleted"=FALSE, "fIndexed"=FALSE, "fFreeList"=FALSE}, {"ixField"=0, "iSequenceOrder"=0, "sxFieldId"="IM25_Frequency_Average", "sxSequenceId"="", "sDisplayName"="IM25 Frequency Average", "sValue"="0", "sUnits"="MHz", "nDataType"=enum."numeric", "nNextItem"=enum."Reset", "fSystem"=TRUE, "fSystemValue"=TRUE, "fRequired"=TRUE, "fSetAtTest"=TRUE, "fTestField"=TRUE, "fDeleted"=FALSE, "fIndexed"=FALSE, "fFreeList"=FALSE}, {"ixField"=0, "iSequenceOrder"=0, "sxFieldId"="IM25_Frequency_Maximum", "sxSequenceId"="", "sDisplayName"="IM25 Frequency Maximum", "sValue"="0", "sUnits"="MHz", "nDataType"=enum."numeric", "nNextItem"=enum."Reset", "fSystem"=TRUE, "fSystemValue"=TRUE, "fRequired"=TRUE, "fSetAtTest"=TRUE, "fTestField"=TRUE, "fDeleted"=FALSE, "fIndexed"=FALSE, "fFreeList"=FALSE}, {"ixField"=0, "iSequenceOrder"=0, "sxFieldId"="IM25_Frequency_Minimum", "sxSequenceId"="", "sDisplayName"="IM25 Frequency Minimum", "sValue"="0", "sUnits"="MHz", "nDataType"=enum."numeric", "nNextItem"=enum."Reset", "fSystem"=TRUE, "fSystemValue"=TRUE, "fRequired"=TRUE, "fSetAtTest"=TRUE, "fTestField"=TRUE, "fDeleted"=FALSE, "fIndexed"=FALSE, "fFreeList"=FALSE}, {"ixField"=0, "iSequenceOrder"=0, "sxFieldId"="IM25_Frequency_Standard_Deviation", "sxSequenceId"="", "sDisplayName"="IM25 Frequency Standard Deviation", "sValue"="0", "sUnits"="MHz", "nDataType"=enum."numeric", "nNextItem"=enum."Reset", "fSystem"=TRUE, "fSystemValue"=TRUE, "fRequired"=TRUE, "fSetAtTest"=TRUE, "fTestField"=TRUE, "fDeleted"=FALSE, "fIndexed"=FALSE, "fFreeList"=FALSE}, {"ixField"=0, "iSequenceOrder"=0, "sxFieldId"="IM25_Power_1_Average", "sxSequenceId"="", "sDisplayName"="IM25 Power 1 Average", "sValue"="0", "sUnits"="dBm", "nDataType"=enum."numeric", "nNextItem"=enum."Reset", "fSystem"=TRUE, "fSystemValue"=TRUE, "fRequired"=TRUE, "fSetAtTest"=TRUE, "fTestField"=TRUE, "fDeleted"=FALSE, "fIndexed"=FALSE, "fFreeList"=FALSE}, {"ixField"=0, "iSequenceOrder"=0, "sxFieldId"="IM25_Power_1_Maximum", "sxSequenceId"="", "sDisplayName"="IM25 Power 1 Maximum", "sValue"="0", "sUnits"="dBm", "nDataType"=enum."numeric", "nNextItem"=enum."Reset", "fSystem"=TRUE, "fSystemValue"=TRUE, "fRequired"=TRUE, "fSetAtTest"=TRUE, "fTestField"=TRUE, "fDeleted"=FALSE, "fIndexed"=FALSE, "fFreeList"=FALSE}, {"ixField"=0, "iSequenceOrder"=0, "sxFieldId"="IM25_Power_1_Minimum", "sxSequenceId"="", "sDisplayName"="IM25 Power 1 Minimum", "sValue"="0", "sUnits"="dBm", "nDataType"=enum."numeric", "nNextItem"=enum."Reset", "fSystem"=TRUE, "fSystemValue"=TRUE, "fRequired"=TRUE, "fSetAtTest"=TRUE, "fTestField"=TRUE, "fDeleted"=FALSE, "fIndexed"=FALSE, "fFreeList"=FALSE}, {"ixField"=0, "iSequenceOrder"=0, "sxFieldId"="IM25_Power_1_Standard_Deviation", "sxSequenceId"="", "sDisplayName"="IM25 Power 1 Standard Deviation", "sValue"="0", "sUnits"="dBm", "nDataType"=enum."numeric", "nNextItem"=enum."Reset", "fSystem"=TRUE, "fSystemValue"=TRUE, "fRequired"=TRUE, "fSetAtTest"=TRUE, "fTestField"=TRUE, "fDeleted"=FALSE, "fIndexed"=FALSE, "fFreeList"=FALSE}, {"ixField"=0, "iSequenceOrder"=0, "sxFieldId"="IM25_Power_2_Average", "sxSequenceId"="", "sDisplayName"="IM25 Power 2 Average", "sValue"="0", "sUnits"="dBc", "nDataType"=enum."numeric", "nNextItem"=enum."Reset", "fSystem"=TRUE, "fSystemValue"=TRUE, "fRequired"=TRUE, "fSetAtTest"=TRUE, "fTestField"=TRUE, "fDeleted"=FALSE, "fIndexed"=FALSE, "fFreeList"=FALSE}, {"ixField"=0, "iSequenceOrder"=0, "sxFieldId"="IM25_Power_2_Maximum", "sxSequenceId"="", "sDisplayName"="IM25 Power 2 Maximum", "sValue"="0", "sUnits"="dBc", "nDataType"=enum."numeric", "nNextItem"=enum."Reset", "fSystem"=TRUE, "fSystemValue"=TRUE, "fRequired"=TRUE, "fSetAtTest"=TRUE, "fTestField"=TRUE, "fDeleted"=FALSE, "fIndexed"=FALSE, "fFreeList"=FALSE}, {"ixField"=0, "iSequenceOrder"=0, "sxFieldId"="IM25_Power_2_Minimum", "sxSequenceId"="", "sDisplayName"="IM25 Power 2 Minimum", "sValue"="0", "sUnits"="dBc", "nDataType"=enum."numeric", "nNextItem"=enum."Reset", "fSystem"=TRUE, "fSystemValue"=TRUE, "fRequired"=TRUE, "fSetAtTest"=TRUE, "fTestField"=TRUE, "fDeleted"=FALSE, "fIndexed"=FALSE, "fFreeList"=FALSE}, {"ixField"=0, "iSequenceOrder"=0, "sxFieldId"="IM25_Power_2_Standard_Deviation", "sxSequenceId"="", "sDisplayName"="IM25 Power 2 Standard Deviation", "sValue"="0", "sUnits"="dBc", "nDataType"=enum."numeric", "nNextItem"=enum."Reset", "fSystem"=TRUE, "fSystemValue"=TRUE, "fRequired"=TRUE, "fSetAtTest"=TRUE, "fTestField"=TRUE, "fDeleted"=FALSE, "fIndexed"=FALSE, "fFreeList"=FALSE}, {"ixField"=0, "iSequenceOrder"=0, "sxFieldId"="IM27_Frequency_Average", "sxSequenceId"="", "sDisplayName"="IM27 Frequency Average", "sValue"="0", "sUnits"="MHz", "nDataType"=enum."numeric", "nNextItem"=enum."Reset", "fSystem"=TRUE, "fSystemValue"=TRUE, "fRequired"=TRUE, "fSetAtTest"=TRUE, "fTestField"=TRUE, "fDeleted"=FALSE, "fIndexed"=FALSE, "fFreeList"=FALSE}, {"ixField"=0, "iSequenceOrder"=0, "sxFieldId"="IM27_Frequency_Maximum", "sxSequenceId"="", "sDisplayName"="IM27 Frequency Maximum", "sValue"="0", "sUnits"="MHz", "nDataType"=enum."numeric", "nNextItem"=enum."Reset", "fSystem"=TRUE, "fSystemValue"=TRUE, "fRequired"=TRUE, "fSetAtTest"=TRUE, "fTestField"=TRUE, "fDeleted"=FALSE, "fIndexed"=FALSE, "fFreeList"=FALSE}, {"ixField"=0, "iSequenceOrder"=0, "sxFieldId"="IM27_Frequency_Minimum", "sxSequenceId"="", "sDisplayName"="IM27 Frequency Minimum", "sValue"="0", "sUnits"="MHz", "nDataType"=enum."numeric", "nNextItem"=enum."Reset", "fSystem"=TRUE, "fSystemValue"=TRUE, "fRequired"=TRUE, "fSetAtTest"=TRUE, "fTestField"=TRUE, "fDeleted"=FALSE, "fIndexed"=FALSE, "fFreeList"=FALSE}, {"ixField"=0, "iSequenceOrder"=0, "sxFieldId"="IM27_Frequency_Standard_Deviation", "sxSequenceId"="", "sDisplayName"="IM27 Frequency Standard Deviation", "sValue"="0", "sUnits"="MHz", "nDataType"=enum."numeric", "nNextItem"=enum."Reset", "fSystem"=TRUE, "fSystemValue"=TRUE, "fRequired"=TRUE, "fSetAtTest"=TRUE, "fTestField"=TRUE, "fDeleted"=FALSE, "fIndexed"=FALSE, "fFreeList"=FALSE}, {"ixField"=0, "iSequenceOrder"=0, "sxFieldId"="IM27_Power_1_Average", "sxSequenceId"="", "sDisplayName"="IM27 Power 1 Average", "sValue"="0", "sUnits"="dBm", "nDataType"=enum."numeric", "nNextItem"=enum."Reset", "fSystem"=TRUE, "fSystemValue"=TRUE, "fRequired"=TRUE, "fSetAtTest"=TRUE, "fTestField"=TRUE, "fDeleted"=FALSE, "fIndexed"=FALSE, "fFreeList"=FALSE}, {"ixField"=0, "iSequenceOrder"=0, "sxFieldId"="IM27_Power_1_Maximum", "sxSequenceId"="", "sDisplayName"="IM27 Power 1 Maximum", "sValue"="0", "sUnits"="dBm", "nDataType"=enum."numeric", "nNextItem"=enum."Reset", "fSystem"=TRUE, "fSystemValue"=TRUE, "fRequired"=TRUE, "fSetAtTest"=TRUE, "fTestField"=TRUE, "fDeleted"=FALSE, "fIndexed"=FALSE, "fFreeList"=FALSE}, {"ixField"=0, "iSequenceOrder"=0, "sxFieldId"="IM27_Power_1_Minimum", "sxSequenceId"="", "sDisplayName"="IM27 Power 1 Minimum", "sValue"="0", "sUnits"="dBm", "nDataType"=enum."numeric", "nNextItem"=enum."Reset", "fSystem"=TRUE, "fSystemValue"=TRUE, "fRequired"=TRUE, "fSetAtTest"=TRUE, "fTestField"=TRUE, "fDeleted"=FALSE, "fIndexed"=FALSE, "fFreeList"=FALSE}, {"ixField"=0, "iSequenceOrder"=0, "sxFieldId"="IM27_Power_1_Standard_Deviation", "sxSequenceId"="", "sDisplayName"="IM27 Power 1 Standard Deviation", "sValue"="0", "sUnits"="dBm", "nDataType"=enum."numeric", "nNextItem"=enum."Reset", "fSystem"=TRUE, "fSystemValue"=TRUE, "fRequired"=TRUE, "fSetAtTest"=TRUE, "fTestField"=TRUE, "fDeleted"=FALSE, "fIndexed"=FALSE, "fFreeList"=FALSE}, {"ixField"=0, "iSequenceOrder"=0, "sxFieldId"="IM27_Power_2_Average", "sxSequenceId"="", "sDisplayName"="IM27 Power 2 Average", "sValue"="0", "sUnits"="dBc", "nDataType"=enum."numeric", "nNextItem"=enum."Reset", "fSystem"=TRUE, "fSystemValue"=TRUE, "fRequired"=TRUE, "fSetAtTest"=TRUE, "fTestField"=TRUE, "fDeleted"=FALSE, "fIndexed"=FALSE, "fFreeList"=FALSE}, {"ixField"=0, "iSequenceOrder"=0, "sxFieldId"="IM27_Power_2_Maximum", "sxSequenceId"="", "sDisplayName"="IM27 Power 2 Maximum", "sValue"="0", "sUnits"="dBc", "nDataType"=enum."numeric", "nNextItem"=enum."Reset", "fSystem"=TRUE, "fSystemValue"=TRUE, "fRequired"=TRUE, "fSetAtTest"=TRUE, "fTestField"=TRUE, "fDeleted"=FALSE, "fIndexed"=FALSE, "fFreeList"=FALSE}, {"ixField"=0, "iSequenceOrder"=0, "sxFieldId"="IM27_Power_2_Minimum", "sxSequenceId"="", "sDisplayName"="IM27 Power 2 Minimum", "sValue"="0", "sUnits"="dBc", "nDataType"=enum."numeric", "nNextItem"=enum."Reset", "fSystem"=TRUE, "fSystemValue"=TRUE, "fRequired"=TRUE, "fSetAtTest"=TRUE, "fTestField"=TRUE, "fDeleted"=FALSE, "fIndexed"=FALSE, "fFreeList"=FALSE}, {"ixField"=0, "iSequenceOrder"=0, "sxFieldId"="IM27_Power_2_Standard_Deviation", "sxSequenceId"="", "sDisplayName"="IM27 Power 2 Standard Deviation", "sValue"="0", "sUnits"="dBc", "nDataType"=enum."numeric", "nNextItem"=enum."Reset", "fSystem"=TRUE, "fSystemValue"=TRUE, "fRequired"=TRUE, "fSetAtTest"=TRUE, "fTestField"=TRUE, "fDeleted"=FALSE, "fIndexed"=FALSE, "fFreeList"=FALSE}, {"ixField"=0, "iSequenceOrder"=0, "sxFieldId"="IM29_Frequency_Average", "sxSequenceId"="", "sDisplayName"="IM29 Frequency Average", "sValue"="0", "sUnits"="MHz", "nDataType"=enum."numeric", "nNextItem"=enum."Reset", "fSystem"=TRUE, "fSystemValue"=TRUE, "fRequired"=TRUE, "fSetAtTest"=TRUE, "fTestField"=TRUE, "fDeleted"=FALSE, "fIndexed"=FALSE, "fFreeList"=FALSE}, {"ixField"=0, "iSequenceOrder"=0, "sxFieldId"="IM29_Frequency_Maximum", "sxSequenceId"="", "sDisplayName"="IM29 Frequency Maximum", "sValue"="0", "sUnits"="MHz", "nDataType"=enum."numeric", "nNextItem"=enum."Reset", "fSystem"=TRUE, "fSystemValue"=TRUE, "fRequired"=TRUE, "fSetAtTest"=TRUE, "fTestField"=TRUE, "fDeleted"=FALSE, "fIndexed"=FALSE, "fFreeList"=FALSE}, {"ixField"=0, "iSequenceOrder"=0, "sxFieldId"="IM29_Frequency_Minimum", "sxSequenceId"="", "sDisplayName"="IM29 Frequency Minimum", "sValue"="0", "sUnits"="MHz", "nDataType"=enum."numeric", "nNextItem"=enum."Reset", "fSystem"=TRUE, "fSystemValue"=TRUE, "fRequired"=TRUE, "fSetAtTest"=TRUE, "fTestField"=TRUE, "fDeleted"=FALSE, "fIndexed"=FALSE, "fFreeList"=FALSE}, {"ixField"=0, "iSequenceOrder"=0, "sxFieldId"="IM29_Frequency_Standard_Deviation", "sxSequenceId"="", "sDisplayName"="IM29 Frequency Standard Deviation", "sValue"="0", "sUnits"="MHz", "nDataType"=enum."numeric", "nNextItem"=enum."Reset", "fSystem"=TRUE, "fSystemValue"=TRUE, "fRequired"=TRUE, "fSetAtTest"=TRUE, "fTestField"=TRUE, "fDeleted"=FALSE, "fIndexed"=FALSE, "fFreeList"=FALSE}, {"ixField"=0, "iSequenceOrder"=0, "sxFieldId"="IM29_Power_1_Average", "sxSequenceId"="", "sDisplayName"="IM29 Power 1 Average", "sValue"="0", "sUnits"="dBm", "nDataType"=enum."numeric", "nNextItem"=enum."Reset", "fSystem"=TRUE, "fSystemValue"=TRUE, "fRequired"=TRUE, "fSetAtTest"=TRUE, "fTestField"=TRUE, "fDeleted"=FALSE, "fIndexed"=FALSE, "fFreeList"=FALSE}, {"ixField"=0, "iSequenceOrder"=0, "sxFieldId"="IM29_Power_1_Maximum", "sxSequenceId"="", "sDisplayName"="IM29 Power 1 Maximum", "sValue"="0", "sUnits"="dBm", "nDataType"=enum."numeric", "nNextItem"=enum."Reset", "fSystem"=TRUE, "fSystemValue"=TRUE, "fRequired"=TRUE, "fSetAtTest"=TRUE, "fTestField"=TRUE, "fDeleted"=FALSE, "fIndexed"=FALSE, "fFreeList"=FALSE}, {"ixField"=0, "iSequenceOrder"=0, "sxFieldId"="IM29_Power_1_Minimum", "sxSequenceId"="", "sDisplayName"="IM29 Power 1 Minimum", "sValue"="0", "sUnits"="dBm", "nDataType"=enum."numeric", "nNextItem"=enum."Reset", "fSystem"=TRUE, "fSystemValue"=TRUE, "fRequired"=TRUE, "fSetAtTest"=TRUE, "fTestField"=TRUE, "fDeleted"=FALSE, "fIndexed"=FALSE, "fFreeList"=FALSE}, {"ixField"=0, "iSequenceOrder"=0, "sxFieldId"="IM29_Power_1_Standard_Deviation", "sxSequenceId"="", "sDisplayName"="IM29 Power 1 Standard Deviation", "sValue"="0", "sUnits"="dBm", "nDataType"=enum."numeric", "nNextItem"=enum."Reset", "fSystem"=TRUE, "fSystemValue"=TRUE, "fRequired"=TRUE, "fSetAtTest"=TRUE, "fTestField"=TRUE, "fDeleted"=FALSE, "fIndexed"=FALSE, "fFreeList"=FALSE}, {"ixField"=0, "iSequenceOrder"=0, "sxFieldId"="IM29_Power_2_Average", "sxSequenceId"="", "sDisplayName"="IM29 Power 2 Average", "sValue"="0", "sUnits"="dBc", "nDataType"=enum."numeric", "nNextItem"=enum."Reset", "fSystem"=TRUE, "fSystemValue"=TRUE, "fRequired"=TRUE, "fSetAtTest"=TRUE, "fTestField"=TRUE, "fDeleted"=FALSE, "fIndexed"=FALSE, "fFreeList"=FALSE}, {"ixField"=0, "iSequenceOrder"=0, "sxFieldId"="IM29_Power_2_Maximum", "sxSequenceId"="", "sDisplayName"="IM29 Power 2 Maximum", "sValue"="0", "sUnits"="dBc", "nDataType"=enum."numeric", "nNextItem"=enum."Reset", "fSystem"=TRUE, "fSystemValue"=TRUE, "fRequired"=TRUE, "fSetAtTest"=TRUE, "fTestField"=TRUE, "fDeleted"=FALSE, "fIndexed"=FALSE, "fFreeList"=FALSE}, {"ixField"=0, "iSequenceOrder"=0, "sxFieldId"="IM29_Power_2_Minimum", "sxSequenceId"="", "sDisplayName"="IM29 Power 2 Minimum", "sValue"="0", "sUnits"="dBc", "nDataType"=enum."numeric", "nNextItem"=enum."Reset", "fSystem"=TRUE, "fSystemValue"=TRUE, "fRequired"=TRUE, "fSetAtTest"=TRUE, "fTestField"=TRUE, "fDeleted"=FALSE, "fIndexed"=FALSE, "fFreeList"=FALSE}, {"ixField"=0, "iSequenceOrder"=0, "sxFieldId"="IM29_Power_2_Standard_Deviation", "sxSequenceId"="", "sDisplayName"="IM29 Power 2 Standard Deviation", "sValue"="0", "sUnits"="dBc", "nDataType"=enum."numeric", "nNextItem"=enum."Reset", "fSystem"=TRUE, "fSystemValue"=TRUE, "fRequired"=TRUE, "fSetAtTest"=TRUE, "fTestField"=TRUE, "fDeleted"=FALSE, "fIndexed"=FALSE, "fFreeList"=FALSE}, {"ixField"=0, "iSequenceOrder"=0, "sxFieldId"="IM31_Frequency_Average", "sxSequenceId"="", "sDisplayName"="IM31 Frequency Average", "sValue"="0", "sUnits"="MHz", "nDataType"=enum."numeric", "nNextItem"=enum."Reset", "fSystem"=TRUE, "fSystemValue"=TRUE, "fRequired"=TRUE, "fSetAtTest"=TRUE, "fTestField"=TRUE, "fDeleted"=FALSE, "fIndexed"=FALSE, "fFreeList"=FALSE}, {"ixField"=0, "iSequenceOrder"=0, "sxFieldId"="IM31_Frequency_Maximum", "sxSequenceId"="", "sDisplayName"="IM31 Frequency Maximum", "sValue"="0", "sUnits"="MHz", "nDataType"=enum."numeric", "nNextItem"=enum."Reset", "fSystem"=TRUE, "fSystemValue"=TRUE, "fRequired"=TRUE, "fSetAtTest"=TRUE, "fTestField"=TRUE, "fDeleted"=FALSE, "fIndexed"=FALSE, "fFreeList"=FALSE}, {"ixField"=0, "iSequenceOrder"=0, "sxFieldId"="IM31_Frequency_Minimum", "sxSequenceId"="", "sDisplayName"="IM31 Frequency Minimum", "sValue"="0", "sUnits"="MHz", "nDataType"=enum."numeric", "nNextItem"=enum."Reset", "fSystem"=TRUE, "fSystemValue"=TRUE, "fRequired"=TRUE, "fSetAtTest"=TRUE, "fTestField"=TRUE, "fDeleted"=FALSE, "fIndexed"=FALSE, "fFreeList"=FALSE}, {"ixField"=0, "iSequenceOrder"=0, "sxFieldId"="IM31_Frequency_Standard_Deviation", "sxSequenceId"="", "sDisplayName"="IM31 Frequency Standard Deviation", "sValue"="0", "sUnits"="MHz", "nDataType"=enum."numeric", "nNextItem"=enum."Reset", "fSystem"=TRUE, "fSystemValue"=TRUE, "fRequired"=TRUE, "fSetAtTest"=TRUE, "fTestField"=TRUE, "fDeleted"=FALSE, "fIndexed"=FALSE, "fFreeList"=FALSE}, {"ixField"=0, "iSequenceOrder"=0, "sxFieldId"="IM31_Power_1_Average", "sxSequenceId"="", "sDisplayName"="IM31 Power 1 Average", "sValue"="0", "sUnits"="dBm", "nDataType"=enum."numeric", "nNextItem"=enum."Reset", "fSystem"=TRUE, "fSystemValue"=TRUE, "fRequired"=TRUE, "fSetAtTest"=TRUE, "fTestField"=TRUE, "fDeleted"=FALSE, "fIndexed"=FALSE, "fFreeList"=FALSE}, {"ixField"=0, "iSequenceOrder"=0, "sxFieldId"="IM31_Power_1_Maximum", "sxSequenceId"="", "sDisplayName"="IM31 Power 1 Maximum", "sValue"="0", "sUnits"="dBm", "nDataType"=enum."numeric", "nNextItem"=enum."Reset", "fSystem"=TRUE, "fSystemValue"=TRUE, "fRequired"=TRUE, "fSetAtTest"=TRUE, "fTestField"=TRUE, "fDeleted"=FALSE, "fIndexed"=FALSE, "fFreeList"=FALSE}, {"ixField"=0, "iSequenceOrder"=0, "sxFieldId"="IM31_Power_1_Minimum", "sxSequenceId"="", "sDisplayName"="IM31 Power 1 Minimum", "sValue"="0", "sUnits"="dBm", "nDataType"=enum."numeric", "nNextItem"=enum."Reset", "fSystem"=TRUE, "fSystemValue"=TRUE, "fRequired"=TRUE, "fSetAtTest"=TRUE, "fTestField"=TRUE, "fDeleted"=FALSE, "fIndexed"=FALSE, "fFreeList"=FALSE}, {"ixField"=0, "iSequenceOrder"=0, "sxFieldId"="IM31_Power_1_Standard_Deviation", "sxSequenceId"="", "sDisplayName"="IM31 Power 1 Standard Deviation", "sValue"="0", "sUnits"="dBm", "nDataType"=enum."numeric", "nNextItem"=enum."Reset", "fSystem"=TRUE, "fSystemValue"=TRUE, "fRequired"=TRUE, "fSetAtTest"=TRUE, "fTestField"=TRUE, "fDeleted"=FALSE, "fIndexed"=FALSE, "fFreeList"=FALSE}, {"ixField"=0, "iSequenceOrder"=0, "sxFieldId"="IM31_Power_2_Average", "sxSequenceId"="", "sDisplayName"="IM31 Power 2 Average", "sValue"="0", "sUnits"="dBc", "nDataType"=enum."numeric", "nNextItem"=enum."Reset", "fSystem"=TRUE, "fSystemValue"=TRUE, "fRequired"=TRUE, "fSetAtTest"=TRUE, "fTestField"=TRUE, "fDeleted"=FALSE, "fIndexed"=FALSE, "fFreeList"=FALSE}, {"ixField"=0, "iSequenceOrder"=0, "sxFieldId"="IM31_Power_2_Maximum", "sxSequenceId"="", "sDisplayName"="IM31 Power 2 Maximum", "sValue"="0", "sUnits"="dBc", "nDataType"=enum."numeric", "nNextItem"=enum."Reset", "fSystem"=TRUE, "fSystemValue"=TRUE, "fRequired"=TRUE, "fSetAtTest"=TRUE, "fTestField"=TRUE, "fDeleted"=FALSE, "fIndexed"=FALSE, "fFreeList"=FALSE}, {"ixField"=0, "iSequenceOrder"=0, "sxFieldId"="IM31_Power_2_Minimum", "sxSequenceId"="", "sDisplayName"="IM31 Power 2 Minimum", "sValue"="0", "sUnits"="dBc", "nDataType"=enum."numeric", "nNextItem"=enum."Reset", "fSystem"=TRUE, "fSystemValue"=TRUE, "fRequired"=TRUE, "fSetAtTest"=TRUE, "fTestField"=TRUE, "fDeleted"=FALSE, "fIndexed"=FALSE, "fFreeList"=FALSE}, {"ixField"=0, "iSequenceOrder"=0, "sxFieldId"="IM31_Power_2_Standard_Deviation", "sxSequenceId"="", "sDisplayName"="IM31 Power 2 Standard Deviation", "sValue"="0", "sUnits"="dBc", "nDataType"=enum."numeric", "nNextItem"=enum."Reset", "fSystem"=TRUE, "fSystemValue"=TRUE, "fRequired"=TRUE, "fSetAtTest"=TRUE, "fTestField"=TRUE, "fDeleted"=FALSE, "fIndexed"=FALSE, "fFreeList"=FALSE}, {"ixField"=0, "iSequenceOrder"=0, "sxFieldId"="IM33_Frequency_Average", "sxSequenceId"="", "sDisplayName"="IM33 Frequency Average", "sValue"="0", "sUnits"="MHz", "nDataType"=enum."numeric", "nNextItem"=enum."Reset", "fSystem"=TRUE, "fSystemValue"=TRUE, "fRequired"=TRUE, "fSetAtTest"=TRUE, "fTestField"=TRUE, "fDeleted"=FALSE, "fIndexed"=FALSE, "fFreeList"=FALSE}, {"ixField"=0, "iSequenceOrder"=0, "sxFieldId"="IM33_Frequency_Maximum", "sxSequenceId"="", "sDisplayName"="IM33 Frequency Maximum", "sValue"="0", "sUnits"="MHz", "nDataType"=enum."numeric", "nNextItem"=enum."Reset", "fSystem"=TRUE, "fSystemValue"=TRUE, "fRequired"=TRUE, "fSetAtTest"=TRUE, "fTestField"=TRUE, "fDeleted"=FALSE, "fIndexed"=FALSE, "fFreeList"=FALSE}, {"ixField"=0, "iSequenceOrder"=0, "sxFieldId"="IM33_Frequency_Minimum", "sxSequenceId"="", "sDisplayName"="IM33 Frequency Minimum", "sValue"="0", "sUnits"="MHz", "nDataType"=enum."numeric", "nNextItem"=enum."Reset", "fSystem"=TRUE, "fSystemValue"=TRUE, "fRequired"=TRUE, "fSetAtTest"=TRUE, "fTestField"=TRUE, "fDeleted"=FALSE, "fIndexed"=FALSE, "fFreeList"=FALSE}, {"ixField"=0, "iSequenceOrder"=0, "sxFieldId"="IM33_Frequency_Standard_Deviation", "sxSequenceId"="", "sDisplayName"="IM33 Frequency Standard Deviation", "sValue"="0", "sUnits"="MHz", "nDataType"=enum."numeric", "nNextItem"=enum."Reset", "fSystem"=TRUE, "fSystemValue"=TRUE, "fRequired"=TRUE, "fSetAtTest"=TRUE, "fTestField"=TRUE, "fDeleted"=FALSE, "fIndexed"=FALSE, "fFreeList"=FALSE}, {"ixField"=0, "iSequenceOrder"=0, "sxFieldId"="IM33_Power_1_Average", "sxSequenceId"="", "sDisplayName"="IM33 Power 1 Average", "sValue"="0", "sUnits"="dBm", "nDataType"=enum."numeric", "nNextItem"=enum."Reset", "fSystem"=TRUE, "fSystemValue"=TRUE, "fRequired"=TRUE, "fSetAtTest"=TRUE, "fTestField"=TRUE, "fDeleted"=FALSE, "fIndexed"=FALSE, "fFreeList"=FALSE}, {"ixField"=0, "iSequenceOrder"=0, "sxFieldId"="IM33_Power_1_Maximum", "sxSequenceId"="", "sDisplayName"="IM33 Power 1 Maximum", "sValue"="0", "sUnits"="dBm", "nDataType"=enum."numeric", "nNextItem"=enum."Reset", "fSystem"=TRUE, "fSystemValue"=TRUE, "fRequired"=TRUE, "fSetAtTest"=TRUE, "fTestField"=TRUE, "fDeleted"=FALSE, "fIndexed"=FALSE, "fFreeList"=FALSE}, {"ixField"=0, "iSequenceOrder"=0, "sxFieldId"="IM33_Power_1_Minimum", "sxSequenceId"="", "sDisplayName"="IM33 Power 1 Minimum", "sValue"="0", "sUnits"="dBm", "nDataType"=enum."numeric", "nNextItem"=enum."Reset", "fSystem"=TRUE, "fSystemValue"=TRUE, "fRequired"=TRUE, "fSetAtTest"=TRUE, "fTestField"=TRUE, "fDeleted"=FALSE, "fIndexed"=FALSE, "fFreeList"=FALSE}, {"ixField"=0, "iSequenceOrder"=0, "sxFieldId"="IM33_Power_1_Standard_Deviation", "sxSequenceId"="", "sDisplayName"="IM33 Power 1 Standard Deviation", "sValue"="0", "sUnits"="dBm", "nDataType"=enum."numeric", "nNextItem"=enum."Reset", "fSystem"=TRUE, "fSystemValue"=TRUE, "fRequired"=TRUE, "fSetAtTest"=TRUE, "fTestField"=TRUE, "fDeleted"=FALSE, "fIndexed"=FALSE, "fFreeList"=FALSE}, {"ixField"=0, "iSequenceOrder"=0, "sxFieldId"="IM33_Power_2_Average", "sxSequenceId"="", "sDisplayName"="IM33 Power 2 Average", "sValue"="0", "sUnits"="dBc", "nDataType"=enum."numeric", "nNextItem"=enum."Reset", "fSystem"=TRUE, "fSystemValue"=TRUE, "fRequired"=TRUE, "fSetAtTest"=TRUE, "fTestField"=TRUE, "fDeleted"=FALSE, "fIndexed"=FALSE, "fFreeList"=FALSE}, {"ixField"=0, "iSequenceOrder"=0, "sxFieldId"="IM33_Power_2_Maximum", "sxSequenceId"="", "sDisplayName"="IM33 Power 2 Maximum", "sValue"="0", "sUnits"="dBc", "nDataType"=enum."numeric", "nNextItem"=enum."Reset", "fSystem"=TRUE, "fSystemValue"=TRUE, "fRequired"=TRUE, "fSetAtTest"=TRUE, "fTestField"=TRUE, "fDeleted"=FALSE, "fIndexed"=FALSE, "fFreeList"=FALSE}, {"ixField"=0, "iSequenceOrder"=0, "sxFieldId"="IM33_Power_2_Minimum", "sxSequenceId"="", "sDisplayName"="IM33 Power 2 Minimum", "sValue"="0", "sUnits"="dBc", "nDataType"=enum."numeric", "nNextItem"=enum."Reset", "fSystem"=TRUE, "fSystemValue"=TRUE, "fRequired"=TRUE, "fSetAtTest"=TRUE, "fTestField"=TRUE, "fDeleted"=FALSE, "fIndexed"=FALSE, "fFreeList"=FALSE}, {"ixField"=0, "iSequenceOrder"=0, "sxFieldId"="IM33_Power_2_Standard_Deviation", "sxSequenceId"="", "sDisplayName"="IM33 Power 2 Standard Deviation", "sValue"="0", "sUnits"="dBc", "nDataType"=enum."numeric", "nNextItem"=enum."Reset", "fSystem"=TRUE, "fSystemValue"=TRUE, "fRequired"=TRUE, "fSetAtTest"=TRUE, "fTestField"=TRUE, "fDeleted"=FALSE, "fIndexed"=FALSE, "fFreeList"=FALSE}, {"ixField"=0, "iSequenceOrder"=0, "sxFieldId"="IM3_Frequency_Average", "sxSequenceId"="", "sDisplayName"="IM3 Frequency Average", "sValue"="0", "sUnits"="MHz", "nDataType"=enum."numeric", "nNextItem"=enum."Reset", "fSystem"=TRUE, "fSystemValue"=TRUE, "fRequired"=TRUE, "fSetAtTest"=TRUE, "fTestField"=TRUE, "fDeleted"=FALSE, "fIndexed"=FALSE, "fFreeList"=FALSE}, {"ixField"=0, "iSequenceOrder"=0, "sxFieldId"="IM3_Frequency_Maximum", "sxSequenceId"="", "sDisplayName"="IM3 Frequency Maximum", "sValue"="0", "sUnits"="MHz", "nDataType"=enum."numeric", "nNextItem"=enum."Reset", "fSystem"=TRUE, "fSystemValue"=TRUE, "fRequired"=TRUE, "fSetAtTest"=TRUE, "fTestField"=TRUE, "fDeleted"=FALSE, "fIndexed"=FALSE, "fFreeList"=FALSE}, {"ixField"=0, "iSequenceOrder"=0, "sxFieldId"="IM3_Frequency_Minimum", "sxSequenceId"="", "sDisplayName"="IM3 Frequency Minimum", "sValue"="0", "sUnits"="MHz", "nDataType"=enum."numeric", "nNextItem"=enum."Reset", "fSystem"=TRUE, "fSystemValue"=TRUE, "fRequired"=TRUE, "fSetAtTest"=TRUE, "fTestField"=TRUE, "fDeleted"=FALSE, "fIndexed"=FALSE, "fFreeList"=FALSE}, {"ixField"=0, "iSequenceOrder"=0, "sxFieldId"="IM3_Frequency_Standard_Deviation", "sxSequenceId"="", "sDisplayName"="IM3 Frequency Standard Deviation", "sValue"="0", "sUnits"="MHz", "nDataType"=enum."numeric", "nNextItem"=enum."Reset", "fSystem"=TRUE, "fSystemValue"=TRUE, "fRequired"=TRUE, "fSetAtTest"=TRUE, "fTestField"=TRUE, "fDeleted"=FALSE, "fIndexed"=FALSE, "fFreeList"=FALSE}, {"ixField"=0, "iSequenceOrder"=0, "sxFieldId"="IM3_Power_1_Average", "sxSequenceId"="", "sDisplayName"="IM3 Power 1 Average", "sValue"="0", "sUnits"="dBm", "nDataType"=enum."numeric", "nNextItem"=enum."Reset", "fSystem"=TRUE, "fSystemValue"=TRUE, "fRequired"=TRUE, "fSetAtTest"=TRUE, "fTestField"=TRUE, "fDeleted"=FALSE, "fIndexed"=FALSE, "fFreeList"=FALSE}, {"ixField"=0, "iSequenceOrder"=0, "sxFieldId"="IM3_Power_1_Maximum", "sxSequenceId"="", "sDisplayName"="IM3 Power 1 Maximum", "sValue"="0", "sUnits"="dBm", "nDataType"=enum."numeric", "nNextItem"=enum."Reset", "fSystem"=TRUE, "fSystemValue"=TRUE, "fRequired"=TRUE, "fSetAtTest"=TRUE, "fTestField"=TRUE, "fDeleted"=FALSE, "fIndexed"=FALSE, "fFreeList"=FALSE}, {"ixField"=0, "iSequenceOrder"=0, "sxFieldId"="IM3_Power_1_Minimum", "sxSequenceId"="", "sDisplayName"="IM3 Power 1 Minimum", "sValue"="0", "sUnits"="dBm", "nDataType"=enum."numeric", "nNextItem"=enum."Reset", "fSystem"=TRUE, "fSystemValue"=TRUE, "fRequired"=TRUE, "fSetAtTest"=TRUE, "fTestField"=TRUE, "fDeleted"=FALSE, "fIndexed"=FALSE, "fFreeList"=FALSE}, {"ixField"=0, "iSequenceOrder"=0, "sxFieldId"="IM3_Power_1_Standard_Deviation", "sxSequenceId"="", "sDisplayName"="IM3 Power 1 Standard Deviation", "sValue"="0", "sUnits"="dBm", "nDataType"=enum."numeric", "nNextItem"=enum."Reset", "fSystem"=TRUE, "fSystemValue"=TRUE, "fRequired"=TRUE, "fSetAtTest"=TRUE, "fTestField"=TRUE, "fDeleted"=FALSE, "fIndexed"=FALSE, "fFreeList"=FALSE}, {"ixField"=0, "iSequenceOrder"=0, "sxFieldId"="IM3_Power_2_Average", "sxSequenceId"="", "sDisplayName"="IM3 Power 2 Average", "sValue"="0", "sUnits"="dBc", "nDataType"=enum."numeric", "nNextItem"=enum."Reset", "fSystem"=TRUE, "fSystemValue"=TRUE, "fRequired"=TRUE, "fSetAtTest"=TRUE, "fTestField"=TRUE, "fDeleted"=FALSE, "fIndexed"=FALSE, "fFreeList"=FALSE}, {"ixField"=0, "iSequenceOrder"=0, "sxFieldId"="IM3_Power_2_Maximum", "sxSequenceId"="", "sDisplayName"="IM3 Power 2 Maximum", "sValue"="0", "sUnits"="dBc", "nDataType"=enum."numeric", "nNextItem"=enum."Reset", "fSystem"=TRUE, "fSystemValue"=TRUE, "fRequired"=TRUE, "fSetAtTest"=TRUE, "fTestField"=TRUE, "fDeleted"=FALSE, "fIndexed"=FALSE, "fFreeList"=FALSE}, {"ixField"=0, "iSequenceOrder"=0, "sxFieldId"="IM3_Power_2_Minimum", "sxSequenceId"="", "sDisplayName"="IM3 Power 2 Minimum", "sValue"="0", "sUnits"="dBc", "nDataType"=enum."numeric", "nNextItem"=enum."Reset", "fSystem"=TRUE, "fSystemValue"=TRUE, "fRequired"=TRUE, "fSetAtTest"=TRUE, "fTestField"=TRUE, "fDeleted"=FALSE, "fIndexed"=FALSE, "fFreeList"=FALSE}, {"ixField"=0, "iSequenceOrder"=0, "sxFieldId"="IM3_Power_2_Standard_Deviation", "sxSequenceId"="", "sDisplayName"="IM3 Power 2 Standard Deviation", "sValue"="0", "sUnits"="dBc", "nDataType"=enum."numeric", "nNextItem"=enum."Reset", "fSystem"=TRUE, "fSystemValue"=TRUE, "fRequired"=TRUE, "fSetAtTest"=TRUE, "fTestField"=TRUE, "fDeleted"=FALSE, "fIndexed"=FALSE, "fFreeList"=FALSE}, {"ixField"=0, "iSequenceOrder"=0, "sxFieldId"="IM5_Frequency_Average", "sxSequenceId"="", "sDisplayName"="IM5 Frequency Average", "sValue"="0", "sUnits"="MHz", "nDataType"=enum."numeric", "nNextItem"=enum."Reset", "fSystem"=TRUE, "fSystemValue"=TRUE, "fRequired"=TRUE, "fSetAtTest"=TRUE, "fTestField"=TRUE, "fDeleted"=FALSE, "fIndexed"=FALSE, "fFreeList"=FALSE}, {"ixField"=0, "iSequenceOrder"=0, "sxFieldId"="IM5_Frequency_Maximum", "sxSequenceId"="", "sDisplayName"="IM5 Frequency Maximum", "sValue"="0", "sUnits"="MHz", "nDataType"=enum."numeric", "nNextItem"=enum."Reset", "fSystem"=TRUE, "fSystemValue"=TRUE, "fRequired"=TRUE, "fSetAtTest"=TRUE, "fTestField"=TRUE, "fDeleted"=FALSE, "fIndexed"=FALSE, "fFreeList"=FALSE}, {"ixField"=0, "iSequenceOrder"=0, "sxFieldId"="IM5_Frequency_Minimum", "sxSequenceId"="", "sDisplayName"="IM5 Frequency Minimum", "sValue"="0", "sUnits"="MHz", "nDataType"=enum."numeric", "nNextItem"=enum."Reset", "fSystem"=TRUE, "fSystemValue"=TRUE, "fRequired"=TRUE, "fSetAtTest"=TRUE, "fTestField"=TRUE, "fDeleted"=FALSE, "fIndexed"=FALSE, "fFreeList"=FALSE}, {"ixField"=0, "iSequenceOrder"=0, "sxFieldId"="IM5_Frequency_Standard_Deviation", "sxSequenceId"="", "sDisplayName"="IM5 Frequency Standard Deviation", "sValue"="0", "sUnits"="MHz", "nDataType"=enum."numeric", "nNextItem"=enum."Reset", "fSystem"=TRUE, "fSystemValue"=TRUE, "fRequired"=TRUE, "fSetAtTest"=TRUE, "fTestField"=TRUE, "fDeleted"=FALSE, "fIndexed"=FALSE, "fFreeList"=FALSE}, {"ixField"=0, "iSequenceOrder"=0, "sxFieldId"="IM5_Power_1_Average", "sxSequenceId"="", "sDisplayName"="IM5 Power 1 Average", "sValue"="0", "sUnits"="dBm", "nDataType"=enum."numeric", "nNextItem"=enum."Reset", "fSystem"=TRUE, "fSystemValue"=TRUE, "fRequired"=TRUE, "fSetAtTest"=TRUE, "fTestField"=TRUE, "fDeleted"=FALSE, "fIndexed"=FALSE, "fFreeList"=FALSE}, {"ixField"=0, "iSequenceOrder"=0, "sxFieldId"="IM5_Power_1_Maximum", "sxSequenceId"="", "sDisplayName"="IM5 Power 1 Maximum", "sValue"="0", "sUnits"="dBm", "nDataType"=enum."numeric", "nNextItem"=enum."Reset", "fSystem"=TRUE, "fSystemValue"=TRUE, "fRequired"=TRUE, "fSetAtTest"=TRUE, "fTestField"=TRUE, "fDeleted"=FALSE, "fIndexed"=FALSE, "fFreeList"=FALSE}, {"ixField"=0, "iSequenceOrder"=0, "sxFieldId"="IM5_Power_1_Minimum", "sxSequenceId"="", "sDisplayName"="IM5 Power 1 Minimum", "sValue"="0", "sUnits"="dBm", "nDataType"=enum."numeric", "nNextItem"=enum."Reset", "fSystem"=TRUE, "fSystemValue"=TRUE, "fRequired"=TRUE, "fSetAtTest"=TRUE, "fTestField"=TRUE, "fDeleted"=FALSE, "fIndexed"=FALSE, "fFreeList"=FALSE}, {"ixField"=0, "iSequenceOrder"=0, "sxFieldId"="IM5_Power_1_Standard_Deviation", "sxSequenceId"="", "sDisplayName"="IM5 Power 1 Standard Deviation", "sValue"="0", "sUnits"="dBm", "nDataType"=enum."numeric", "nNextItem"=enum."Reset", "fSystem"=TRUE, "fSystemValue"=TRUE, "fRequired"=TRUE, "fSetAtTest"=TRUE, "fTestField"=TRUE, "fDeleted"=FALSE, "fIndexed"=FALSE, "fFreeList"=FALSE}, {"ixField"=0, "iSequenceOrder"=0, "sxFieldId"="IM5_Power_2_Average", "sxSequenceId"="", "sDisplayName"="IM5 Power 2 Average", "sValue"="0", "sUnits"="dBc", "nDataType"=enum."numeric", "nNextItem"=enum."Reset", "fSystem"=TRUE, "fSystemValue"=TRUE, "fRequired"=TRUE, "fSetAtTest"=TRUE, "fTestField"=TRUE, "fDeleted"=FALSE, "fIndexed"=FALSE, "fFreeList"=FALSE}, {"ixField"=0, "iSequenceOrder"=0, "sxFieldId"="IM5_Power_2_Maximum", "sxSequenceId"="", "sDisplayName"="IM5 Power 2 Maximum", "sValue"="0", "sUnits"="dBc", "nDataType"=enum."numeric", "nNextItem"=enum."Reset", "fSystem"=TRUE, "fSystemValue"=TRUE, "fRequired"=TRUE, "fSetAtTest"=TRUE, "fTestField"=TRUE, "fDeleted"=FALSE, "fIndexed"=FALSE, "fFreeList"=FALSE}, {"ixField"=0, "iSequenceOrder"=0, "sxFieldId"="IM5_Power_2_Minimum", "sxSequenceId"="", "sDisplayName"="IM5 Power 2 Minimum", "sValue"="0", "sUnits"="dBc", "nDataType"=enum."numeric", "nNextItem"=enum."Reset", "fSystem"=TRUE, "fSystemValue"=TRUE, "fRequired"=TRUE, "fSetAtTest"=TRUE, "fTestField"=TRUE, "fDeleted"=FALSE, "fIndexed"=FALSE, "fFreeList"=FALSE}, {"ixField"=0, "iSequenceOrder"=0, "sxFieldId"="IM5_Power_2_Standard_Deviation", "sxSequenceId"="", "sDisplayName"="IM5 Power 2 Standard Deviation", "sValue"="0", "sUnits"="dBc", "nDataType"=enum."numeric", "nNextItem"=enum."Reset", "fSystem"=TRUE, "fSystemValue"=TRUE, "fRequired"=TRUE, "fSetAtTest"=TRUE, "fTestField"=TRUE, "fDeleted"=FALSE, "fIndexed"=FALSE, "fFreeList"=FALSE}, {"ixField"=0, "iSequenceOrder"=0, "sxFieldId"="IM7_Frequency_Average", "sxSequenceId"="", "sDisplayName"="IM7 Frequency Average", "sValue"="0", "sUnits"="MHz", "nDataType"=enum."numeric", "nNextItem"=enum."Reset", "fSystem"=TRUE, "fSystemValue"=TRUE, "fRequired"=TRUE, "fSetAtTest"=TRUE, "fTestField"=TRUE, "fDeleted"=FALSE, "fIndexed"=FALSE, "fFreeList"=FALSE}, {"ixField"=0, "iSequenceOrder"=0, "sxFieldId"="IM7_Frequency_Maximum", "sxSequenceId"="", "sDisplayName"="IM7 Frequency Maximum", "sValue"="0", "sUnits"="MHz", "nDataType"=enum."numeric", "nNextItem"=enum."Reset", "fSystem"=TRUE, "fSystemValue"=TRUE, "fRequired"=TRUE, "fSetAtTest"=TRUE, "fTestField"=TRUE, "fDeleted"=FALSE, "fIndexed"=FALSE, "fFreeList"=FALSE}, {"ixField"=0, "iSequenceOrder"=0, "sxFieldId"="IM7_Frequency_Minimum", "sxSequenceId"="", "sDisplayName"="IM7 Frequency Minimum", "sValue"="0", "sUnits"="MHz", "nDataType"=enum."numeric", "nNextItem"=enum."Reset", "fSystem"=TRUE, "fSystemValue"=TRUE, "fRequired"=TRUE, "fSetAtTest"=TRUE, "fTestField"=TRUE, "fDeleted"=FALSE, "fIndexed"=FALSE, "fFreeList"=FALSE}, {"ixField"=0, "iSequenceOrder"=0, "sxFieldId"="IM7_Frequency_Standard_Deviation", "sxSequenceId"="", "sDisplayName"="IM7 Frequency Standard Deviation", "sValue"="0", "sUnits"="MHz", "nDataType"=enum."numeric", "nNextItem"=enum."Reset", "fSystem"=TRUE, "fSystemValue"=TRUE, "fRequired"=TRUE, "fSetAtTest"=TRUE, "fTestField"=TRUE, "fDeleted"=FALSE, "fIndexed"=FALSE, "fFreeList"=FALSE}, {"ixField"=0, "iSequenceOrder"=0, "sxFieldId"="IM7_Power_1_Average", "sxSequenceId"="", "sDisplayName"="IM7 Power 1 Average", "sValue"="0", "sUnits"="dBm", "nDataType"=enum."numeric", "nNextItem"=enum."Reset", "fSystem"=TRUE, "fSystemValue"=TRUE, "fRequired"=TRUE, "fSetAtTest"=TRUE, "fTestField"=TRUE, "fDeleted"=FALSE, "fIndexed"=FALSE, "fFreeList"=FALSE}, {"ixField"=0, "iSequenceOrder"=0, "sxFieldId"="IM7_Power_1_Maximum", "sxSequenceId"="", "sDisplayName"="IM7 Power 1 Maximum", "sValue"="0", "sUnits"="dBm", "nDataType"=enum."numeric", "nNextItem"=enum."Reset", "fSystem"=TRUE, "fSystemValue"=TRUE, "fRequired"=TRUE, "fSetAtTest"=TRUE, "fTestField"=TRUE, "fDeleted"=FALSE, "fIndexed"=FALSE, "fFreeList"=FALSE}, {"ixField"=0, "iSequenceOrder"=0, "sxFieldId"="IM7_Power_1_Minimum", "sxSequenceId"="", "sDisplayName"="IM7 Power 1 Minimum", "sValue"="0", "sUnits"="dBm", "nDataType"=enum."numeric", "nNextItem"=enum."Reset", "fSystem"=TRUE, "fSystemValue"=TRUE, "fRequired"=TRUE, "fSetAtTest"=TRUE, "fTestField"=TRUE, "fDeleted"=FALSE, "fIndexed"=FALSE, "fFreeList"=FALSE}, {"ixField"=0, "iSequenceOrder"=0, "sxFieldId"="IM7_Power_1_Standard_Deviation", "sxSequenceId"="", "sDisplayName"="IM7 Power 1 Standard Deviation", "sValue"="0", "sUnits"="dBm", "nDataType"=enum."numeric", "nNextItem"=enum."Reset", "fSystem"=TRUE, "fSystemValue"=TRUE, "fRequired"=TRUE, "fSetAtTest"=TRUE, "fTestField"=TRUE, "fDeleted"=FALSE, "fIndexed"=FALSE, "fFreeList"=FALSE}, {"ixField"=0, "iSequenceOrder"=0, "sxFieldId"="IM7_Power_2_Average", "sxSequenceId"="", "sDisplayName"="IM7 Power 2 Average", "sValue"="0", "sUnits"="dBc", "nDataType"=enum."numeric", "nNextItem"=enum."Reset", "fSystem"=TRUE, "fSystemValue"=TRUE, "fRequired"=TRUE, "fSetAtTest"=TRUE, "fTestField"=TRUE, "fDeleted"=FALSE, "fIndexed"=FALSE, "fFreeList"=FALSE}, {"ixField"=0, "iSequenceOrder"=0, "sxFieldId"="IM7_Power_2_Maximum", "sxSequenceId"="", "sDisplayName"="IM7 Power 2 Maximum", "sValue"="0", "sUnits"="dBc", "nDataType"=enum."numeric", "nNextItem"=enum."Reset", "fSystem"=TRUE, "fSystemValue"=TRUE, "fRequired"=TRUE, "fSetAtTest"=TRUE, "fTestField"=TRUE, "fDeleted"=FALSE, "fIndexed"=FALSE, "fFreeList"=FALSE}, {"ixField"=0, "iSequenceOrder"=0, "sxFieldId"="IM7_Power_2_Minimum", "sxSequenceId"="", "sDisplayName"="IM7 Power 2 Minimum", "sValue"="0", "sUnits"="dBc", "nDataType"=enum."numeric", "nNextItem"=enum."Reset", "fSystem"=TRUE, "fSystemValue"=TRUE, "fRequired"=TRUE, "fSetAtTest"=TRUE, "fTestField"=TRUE, "fDeleted"=FALSE, "fIndexed"=FALSE, "fFreeList"=FALSE}, {"ixField"=0, "iSequenceOrder"=0, "sxFieldId"="IM7_Power_2_Standard_Deviation", "sxSequenceId"="", "sDisplayName"="IM7 Power 2 Standard Deviation", "sValue"="0", "sUnits"="dBc", "nDataType"=enum."numeric", "nNextItem"=enum."Reset", "fSystem"=TRUE, "fSystemValue"=TRUE, "fRequired"=TRUE, "fSetAtTest"=TRUE, "fTestField"=TRUE, "fDeleted"=FALSE, "fIndexed"=FALSE, "fFreeList"=FALSE}, {"ixField"=0, "iSequenceOrder"=0, "sxFieldId"="IM9_Frequency_Average", "sxSequenceId"="", "sDisplayName"="IM9 Frequency Average", "sValue"="0", "sUnits"="MHz", "nDataType"=enum."numeric", "nNextItem"=enum."Reset", "fSystem"=TRUE, "fSystemValue"=TRUE, "fRequired"=TRUE, "fSetAtTest"=TRUE, "fTestField"=TRUE, "fDeleted"=FALSE, "fIndexed"=FALSE, "fFreeList"=FALSE}, {"ixField"=0, "iSequenceOrder"=0, "sxFieldId"="IM9_Frequency_Maximum", "sxSequenceId"="", "sDisplayName"="IM9 Frequency Maximum", "sValue"="0", "sUnits"="MHz", "nDataType"=enum."numeric", "nNextItem"=enum."Reset", "fSystem"=TRUE, "fSystemValue"=TRUE, "fRequired"=TRUE, "fSetAtTest"=TRUE, "fTestField"=TRUE, "fDeleted"=FALSE, "fIndexed"=FALSE, "fFreeList"=FALSE}, {"ixField"=0, "iSequenceOrder"=0, "sxFieldId"="IM9_Frequency_Minimum", "sxSequenceId"="", "sDisplayName"="IM9 Frequency Minimum", "sValue"="0", "sUnits"="MHz", "nDataType"=enum."numeric", "nNextItem"=enum."Reset", "fSystem"=TRUE, "fSystemValue"=TRUE, "fRequired"=TRUE, "fSetAtTest"=TRUE, "fTestField"=TRUE, "fDeleted"=FALSE, "fIndexed"=FALSE, "fFreeList"=FALSE}, {"ixField"=0, "iSequenceOrder"=0, "sxFieldId"="IM9_Frequency_Standard_Deviation", "sxSequenceId"="", "sDisplayName"="IM9 Frequency Standard Deviation", "sValue"="0", "sUnits"="MHz", "nDataType"=enum."numeric", "nNextItem"=enum."Reset", "fSystem"=TRUE, "fSystemValue"=TRUE, "fRequired"=TRUE, "fSetAtTest"=TRUE, "fTestField"=TRUE, "fDeleted"=FALSE, "fIndexed"=FALSE, "fFreeList"=FALSE}, {"ixField"=0, "iSequenceOrder"=0, "sxFieldId"="IM9_Power_1_Average", "sxSequenceId"="", "sDisplayName"="IM9 Power 1 Average", "sValue"="0", "sUnits"="dBm", "nDataType"=enum."numeric", "nNextItem"=enum."Reset", "fSystem"=TRUE, "fSystemValue"=TRUE, "fRequired"=TRUE, "fSetAtTest"=TRUE, "fTestField"=TRUE, "fDeleted"=FALSE, "fIndexed"=FALSE, "fFreeList"=FALSE}, {"ixField"=0, "iSequenceOrder"=0, "sxFieldId"="IM9_Power_1_Maximum", "sxSequenceId"="", "sDisplayName"="IM9 Power 1 Maximum", "sValue"="0", "sUnits"="dBm", "nDataType"=enum."numeric", "nNextItem"=enum."Reset", "fSystem"=TRUE, "fSystemValue"=TRUE, "fRequired"=TRUE, "fSetAtTest"=TRUE, "fTestField"=TRUE, "fDeleted"=FALSE, "fIndexed"=FALSE, "fFreeList"=FALSE}, {"ixField"=0, "iSequenceOrder"=0, "sxFieldId"="IM9_Power_1_Minimum", "sxSequenceId"="", "sDisplayName"="IM9 Power 1 Minimum", "sValue"="0", "sUnits"="dBm", "nDataType"=enum."numeric", "nNextItem"=enum."Reset", "fSystem"=TRUE, "fSystemValue"=TRUE, "fRequired"=TRUE, "fSetAtTest"=TRUE, "fTestField"=TRUE, "fDeleted"=FALSE, "fIndexed"=FALSE, "fFreeList"=FALSE}, {"ixField"=0, "iSequenceOrder"=0, "sxFieldId"="IM9_Power_1_Standard_Deviation", "sxSequenceId"="", "sDisplayName"="IM9 Power 1 Standard Deviation", "sValue"="0", "sUnits"="dBm", "nDataType"=enum."numeric", "nNextItem"=enum."Reset", "fSystem"=TRUE, "fSystemValue"=TRUE, "fRequired"=TRUE, "fSetAtTest"=TRUE, "fTestField"=TRUE, "fDeleted"=FALSE, "fIndexed"=FALSE, "fFreeList"=FALSE}, {"ixField"=0, "iSequenceOrder"=0, "sxFieldId"="IM9_Power_2_Average", "sxSequenceId"="", "sDisplayName"="IM9 Power 2 Average", "sValue"="0", "sUnits"="dBc", "nDataType"=enum."numeric", "nNextItem"=enum."Reset", "fSystem"=TRUE, "fSystemValue"=TRUE, "fRequired"=TRUE, "fSetAtTest"=TRUE, "fTestField"=TRUE, "fDeleted"=FALSE, "fIndexed"=FALSE, "fFreeList"=FALSE}, {"ixField"=0, "iSequenceOrder"=0, "sxFieldId"="IM9_Power_2_Maximum", "sxSequenceId"="", "sDisplayName"="IM9 Power 2 Maximum", "sValue"="0", "sUnits"="dBc", "nDataType"=enum."numeric", "nNextItem"=enum."Reset", "fSystem"=TRUE, "fSystemValue"=TRUE, "fRequired"=TRUE, "fSetAtTest"=TRUE, "fTestField"=TRUE, "fDeleted"=FALSE, "fIndexed"=FALSE, "fFreeList"=FALSE}, {"ixField"=0, "iSequenceOrder"=0, "sxFieldId"="IM9_Power_2_Minimum", "sxSequenceId"="", "sDisplayName"="IM9 Power 2 Minimum", "sValue"="0", "sUnits"="dBc", "nDataType"=enum."numeric", "nNextItem"=enum."Reset", "fSystem"=TRUE, "fSystemValue"=TRUE, "fRequired"=TRUE, "fSetAtTest"=TRUE, "fTestField"=TRUE, "fDeleted"=FALSE, "fIndexed"=FALSE, "fFreeList"=FALSE}, {"ixField"=0, "iSequenceOrder"=0, "sxFieldId"="IM9_Power_2_Standard_Deviation", "sxSequenceId"="", "sDisplayName"="IM9 Power 2 Standard Deviation", "sValue"="0", "sUnits"="dBc", "nDataType"=enum."numeric", "nNextItem"=enum."Reset", "fSystem"=TRUE, "fSystemValue"=TRUE, "fRequired"=TRUE, "fSetAtTest"=TRUE, "fTestField"=TRUE, "fDeleted"=FALSE, "fIndexed"=FALSE, "fFreeList"=FALSE}, {"ixField"=0, "iSequenceOrder"=0, "sxFieldId"="IM_Mode", "sxSequenceId"="", "sDisplayName"="IM Mode", "sValue"="Reverse\tReverse\tForward\tAuxilary", "sUnits"="", "nDataType"=enum."list", "nNextItem"=enum."Reset", "fSystem"=TRUE, "fSystemValue"=TRUE, "fRequired"=TRUE, "fSetAtTest"=TRUE, "fTestField"=TRUE, "fDeleted"=FALSE, "fIndexed"=FALSE, "fFreeList"=FALSE}, {"ixField"=0, "iSequenceOrder"=0, "sxFieldId"="IM_Order", "sxSequenceId"="", "sDisplayName"="IM Order", "sValue"="3rd\t3rd\t5th\t7th\t9th\t11th\t13th\t15th\t17th\t19th\t21st\t23rd\t25th\t27th\t29th\t31st\t33rd", "sUnits"="", "nDataType"=enum."list", "nNextItem"=enum."Reset", "fSystem"=TRUE, "fSystemValue"=TRUE, "fRequired"=TRUE, "fSetAtTest"=TRUE, "fTestField"=TRUE, "fDeleted"=FALSE, "fIndexed"=FALSE, "fFreeList"=FALSE}, {"ixField"=0, "iSequenceOrder"=0, "sxFieldId"="Instrument_Calibration_Date", "sxSequenceId"="", "sDisplayName"="Instrument Calibration Date", "sValue"="0", "sUnits"="", "nDataType"=enum."timestamp", "nNextItem"=enum."Reset", "fSystem"=TRUE, "fSystemValue"=TRUE, "fRequired"=TRUE, "fSetAtTest"=TRUE, "fTestField"=TRUE, "fDeleted"=FALSE, "fIndexed"=FALSE, "fFreeList"=FALSE}, {"ixField"=0, "iSequenceOrder"=0, "sxFieldId"="Instrument_Calibration_Due_Date", "sxSequenceId"="", "sDisplayName"="Instrument Calibration Due Date", "sValue"="0", "sUnits"="", "nDataType"=enum."timestamp", "nNextItem"=enum."Reset", "fSystem"=TRUE, "fSystemValue"=TRUE, "fRequired"=TRUE, "fSetAtTest"=TRUE, "fTestField"=TRUE, "fDeleted"=FALSE, "fIndexed"=FALSE, "fFreeList"=FALSE}, {"ixField"=0, "iSequenceOrder"=0, "sxFieldId"="Instrument_Devices_Used", "sxSequenceId"="", "sDisplayName"="Instrument Devices Used", "sValue"="", "sUnits"="", "nDataType"=enum."text", "nNextItem"=enum."Reset", "fSystem"=TRUE, "fSystemValue"=TRUE, "fRequired"=TRUE, "fSetAtTest"=TRUE, "fTestField"=TRUE, "fDeleted"=FALSE, "fIndexed"=FALSE, "fFreeList"=FALSE}, {"ixField"=0, "iSequenceOrder"=0, "sxFieldId"="Instrument_Driver", "sxSequenceId"="", "sDisplayName"="Instrument Driver", "sValue"="", "sUnits"="", "nDataType"=enum."text", "nNextItem"=enum."Reset", "fSystem"=TRUE, "fSystemValue"=TRUE, "fRequired"=TRUE, "fSetAtTest"=TRUE, "fTestField"=TRUE, "fDeleted"=FALSE, "fIndexed"=FALSE, "fFreeList"=FALSE}, {"ixField"=0, "iSequenceOrder"=0, "sxFieldId"="Instrument_Name", "sxSequenceId"="", "sDisplayName"="Instrument Name", "sValue"="", "sUnits"="", "nDataType"=enum."text", "nNextItem"=enum."Reset", "fSystem"=TRUE, "fSystemValue"=TRUE, "fRequired"=TRUE, "fSetAtTest"=TRUE, "fTestField"=TRUE, "fDeleted"=FALSE, "fIndexed"=FALSE, "fFreeList"=FALSE}, {"ixField"=0, "iSequenceOrder"=0, "sxFieldId"="Instrument_Serial_Number", "sxSequenceId"="", "sDisplayName"="Instrument Serial Number", "sValue"="", "sUnits"="", "nDataType"=enum."text", "nNextItem"=enum."Reset", "fSystem"=TRUE, "fSystemValue"=TRUE, "fRequired"=TRUE, "fSetAtTest"=TRUE, "fTestField"=TRUE, "fDeleted"=FALSE, "fIndexed"=FALSE, "fFreeList"=FALSE}, {"ixField"=0, "iSequenceOrder"=0, "sxFieldId"="Instrument_Type", "sxSequenceId"="", "sDisplayName"="Instrument Type", "sValue"="", "sUnits"="", "nDataType"=enum."text", "nNextItem"=enum."Reset", "fSystem"=TRUE, "fSystemValue"=TRUE, "fRequired"=TRUE, "fSetAtTest"=TRUE, "fTestField"=TRUE, "fDeleted"=FALSE, "fIndexed"=FALSE, "fFreeList"=FALSE}, {"ixField"=0, "iSequenceOrder"=0, "sxFieldId"="Measurement_Type", "sxSequenceId"="", "sDisplayName"="Measurement Type", "sValue"="Band Edges\tBand Edges\tFixed Pair\tSwept Freq", "sUnits"="", "nDataType"=enum."list", "nNextItem"=enum."Reset", "fSystem"=TRUE, "fSystemValue"=TRUE, "fRequired"=TRUE, "fSetAtTest"=TRUE, "fTestField"=TRUE, "fDeleted"=FALSE, "fIndexed"=FALSE, "fFreeList"=FALSE}, {"ixField"=0, "iSequenceOrder"=0, "sxFieldId"="Peak_Hold", "sxSequenceId"="", "sDisplayName"="Peak Hold", "sValue"="0", "sUnits"="", "nDataType"=enum."numeric", "nNextItem"=enum."Reset", "fSystem"=TRUE, "fSystemValue"=TRUE, "fRequired"=TRUE, "fSetAtTest"=TRUE, "fTestField"=TRUE, "fDeleted"=FALSE, "fIndexed"=FALSE, "fFreeList"=FALSE}, {"ixField"=0, "iSequenceOrder"=0, "sxFieldId"="Peak_IM_Level", "sxSequenceId"="", "sDisplayName"="Peak IM Level", "sValue"="0", "sUnits"="dBm", "nDataType"=enum."numeric", "nNextItem"=enum."Reset", "fSystem"=TRUE, "fSystemValue"=TRUE, "fRequired"=TRUE, "fSetAtTest"=TRUE, "fTestField"=TRUE, "fDeleted"=FALSE, "fIndexed"=FALSE, "fFreeList"=FALSE}, {"ixField"=0, "iSequenceOrder"=0, "sxFieldId"="Peak_N_Samples", "sxSequenceId"="", "sDisplayName"="Peak N Samples", "sValue"="0", "sUnits"="Samples", "nDataType"=enum."numeric", "nNextItem"=enum."Reset", "fSystem"=TRUE, "fSystemValue"=TRUE, "fRequired"=TRUE, "fSetAtTest"=TRUE, "fTestField"=TRUE, "fDeleted"=FALSE, "fIndexed"=FALSE, "fFreeList"=FALSE}, {"ixField"=0, "iSequenceOrder"=0, "sxFieldId"="Tx1_Frequency_Average", "sxSequenceId"="", "sDisplayName"="Tx1 Frequency Average", "sValue"="0", "sUnits"="MHz", "nDataType"=enum."numeric", "nNextItem"=enum."Reset", "fSystem"=TRUE, "fSystemValue"=TRUE, "fRequired"=TRUE, "fSetAtTest"=TRUE, "fTestField"=TRUE, "fDeleted"=FALSE, "fIndexed"=FALSE, "fFreeList"=FALSE}, {"ixField"=0, "iSequenceOrder"=0, "sxFieldId"="Tx1_Frequency_Maximum", "sxSequenceId"="", "sDisplayName"="Tx1 Frequency Maximum", "sValue"="0", "sUnits"="MHz", "nDataType"=enum."numeric", "nNextItem"=enum."Reset", "fSystem"=TRUE, "fSystemValue"=TRUE, "fRequired"=TRUE, "fSetAtTest"=TRUE, "fTestField"=TRUE, "fDeleted"=FALSE, "fIndexed"=FALSE, "fFreeList"=FALSE}, {"ixField"=0, "iSequenceOrder"=0, "sxFieldId"="Tx1_Frequency_Minimum", "sxSequenceId"="", "sDisplayName"="Tx1 Frequency Minimum", "sValue"="0", "sUnits"="MHz", "nDataType"=enum."numeric", "nNextItem"=enum."Reset", "fSystem"=TRUE, "fSystemValue"=TRUE, "fRequired"=TRUE, "fSetAtTest"=TRUE, "fTestField"=TRUE, "fDeleted"=FALSE, "fIndexed"=FALSE, "fFreeList"=FALSE}, {"ixField"=0, "iSequenceOrder"=0, "sxFieldId"="Tx1_Frequency_Standard_Deviation", "sxSequenceId"="", "sDisplayName"="Tx1 Frequency Standard Deviation", "sValue"="0", "sUnits"="MHz", "nDataType"=enum."numeric", "nNextItem"=enum."Reset", "fSystem"=TRUE, "fSystemValue"=TRUE, "fRequired"=TRUE, "fSetAtTest"=TRUE, "fTestField"=TRUE, "fDeleted"=FALSE, "fIndexed"=FALSE, "fFreeList"=FALSE}, {"ixField"=0, "iSequenceOrder"=0, "sxFieldId"="Tx1_Power_Average", "sxSequenceId"="", "sDisplayName"="Tx1 Power Average", "sValue"="0", "sUnits"="dBm", "nDataType"=enum."numeric", "nNextItem"=enum."Reset", "fSystem"=TRUE, "fSystemValue"=TRUE, "fRequired"=TRUE, "fSetAtTest"=TRUE, "fTestField"=TRUE, "fDeleted"=FALSE, "fIndexed"=FALSE, "fFreeList"=FALSE}, {"ixField"=0, "iSequenceOrder"=0, "sxFieldId"="Tx1_Power_Maximum", "sxSequenceId"="", "sDisplayName"="Tx1 Power Maximum", "sValue"="0", "sUnits"="dBm", "nDataType"=enum."numeric", "nNextItem"=enum."Reset", "fSystem"=TRUE, "fSystemValue"=TRUE, "fRequired"=TRUE, "fSetAtTest"=TRUE, "fTestField"=TRUE, "fDeleted"=FALSE, "fIndexed"=FALSE, "fFreeList"=FALSE}, {"ixField"=0, "iSequenceOrder"=0, "sxFieldId"="Tx1_Power_Minimum", "sxSequenceId"="", "sDisplayName"="Tx1 Power Minimum", "sValue"="0", "sUnits"="dBm", "nDataType"=enum."numeric", "nNextItem"=enum."Reset", "fSystem"=TRUE, "fSystemValue"=TRUE, "fRequired"=TRUE, "fSetAtTest"=TRUE, "fTestField"=TRUE, "fDeleted"=FALSE, "fIndexed"=FALSE, "fFreeList"=FALSE}, {"ixField"=0, "iSequenceOrder"=0, "sxFieldId"="Tx1_Power_Standard_Deviation", "sxSequenceId"="", "sDisplayName"="Tx1 Power Standard Deviation", "sValue"="0", "sUnits"="dBm", "nDataType"=enum."numeric", "nNextItem"=enum."Reset", "fSystem"=TRUE, "fSystemValue"=TRUE, "fRequired"=TRUE, "fSetAtTest"=TRUE, "fTestField"=TRUE, "fDeleted"=FALSE, "fIndexed"=FALSE, "fFreeList"=FALSE}, {"ixField"=0, "iSequenceOrder"=0, "sxFieldId"="Tx2_Frequency_Average", "sxSequenceId"="", "sDisplayName"="Tx2 Frequency Average", "sValue"="0", "sUnits"="MHz", "nDataType"=enum."numeric", "nNextItem"=enum."Reset", "fSystem"=TRUE, "fSystemValue"=TRUE, "fRequired"=TRUE, "fSetAtTest"=TRUE, "fTestField"=TRUE, "fDeleted"=FALSE, "fIndexed"=FALSE, "fFreeList"=FALSE}, {"ixField"=0, "iSequenceOrder"=0, "sxFieldId"="Tx2_Frequency_Maximum", "sxSequenceId"="", "sDisplayName"="Tx2 Frequency Maximum", "sValue"="0", "sUnits"="MHz", "nDataType"=enum."numeric", "nNextItem"=enum."Reset", "fSystem"=TRUE, "fSystemValue"=TRUE, "fRequired"=TRUE, "fSetAtTest"=TRUE, "fTestField"=TRUE, "fDeleted"=FALSE, "fIndexed"=FALSE, "fFreeList"=FALSE}, {"ixField"=0, "iSequenceOrder"=0, "sxFieldId"="Tx2_Frequency_Minimum", "sxSequenceId"="", "sDisplayName"="Tx2 Frequency Minimum", "sValue"="0", "sUnits"="MHz", "nDataType"=enum."numeric", "nNextItem"=enum."Reset", "fSystem"=TRUE, "fSystemValue"=TRUE, "fRequired"=TRUE, "fSetAtTest"=TRUE, "fTestField"=TRUE, "fDeleted"=FALSE, "fIndexed"=FALSE, "fFreeList"=FALSE}, {"ixField"=0, "iSequenceOrder"=0, "sxFieldId"="Tx2_Frequency_Standard_Deviation", "sxSequenceId"="", "sDisplayName"="Tx2 Frequency Standard Deviation", "sValue"="0", "sUnits"="MHz", "nDataType"=enum."numeric", "nNextItem"=enum."Reset", "fSystem"=TRUE, "fSystemValue"=TRUE, "fRequired"=TRUE, "fSetAtTest"=TRUE, "fTestField"=TRUE, "fDeleted"=FALSE, "fIndexed"=FALSE, "fFreeList"=FALSE}, {"ixField"=0, "iSequenceOrder"=0, "sxFieldId"="Tx2_Power_Average", "sxSequenceId"="", "sDisplayName"="Tx2 Power Average", "sValue"="0", "sUnits"="dBm", "nDataType"=enum."numeric", "nNextItem"=enum."Reset", "fSystem"=TRUE, "fSystemValue"=TRUE, "fRequired"=TRUE, "fSetAtTest"=TRUE, "fTestField"=TRUE, "fDeleted"=FALSE, "fIndexed"=FALSE, "fFreeList"=FALSE}, {"ixField"=0, "iSequenceOrder"=0, "sxFieldId"="Tx2_Power_Maximum", "sxSequenceId"="", "sDisplayName"="Tx2 Power Maximum", "sValue"="0", "sUnits"="dBm", "nDataType"=enum."numeric", "nNextItem"=enum."Reset", "fSystem"=TRUE, "fSystemValue"=TRUE, "fRequired"=TRUE, "fSetAtTest"=TRUE, "fTestField"=TRUE, "fDeleted"=FALSE, "fIndexed"=FALSE, "fFreeList"=FALSE}, {"ixField"=0, "iSequenceOrder"=0, "sxFieldId"="Tx2_Power_Minimum", "sxSequenceId"="", "sDisplayName"="Tx2 Power Minimum", "sValue"="0", "sUnits"="dBm", "nDataType"=enum."numeric", "nNextItem"=enum."Reset", "fSystem"=TRUE, "fSystemValue"=TRUE, "fRequired"=TRUE, "fSetAtTest"=TRUE, "fTestField"=TRUE, "fDeleted"=FALSE, "fIndexed"=FALSE, "fFreeList"=FALSE}, {"ixField"=0, "iSequenceOrder"=0, "sxFieldId"="Tx2_Power_Standard_Deviation", "sxSequenceId"="", "sDisplayName"="Tx2 Power Standard Deviation", "sValue"="0", "sUnits"="dBm", "nDataType"=enum."numeric", "nNextItem"=enum."Reset", "fSystem"=TRUE, "fSystemValue"=TRUE, "fRequired"=TRUE, "fSetAtTest"=TRUE, "fTestField"=TRUE, "fDeleted"=FALSE, "fIndexed"=FALSE, "fFreeList"=FALSE}, {"ixField"=0, "iSequenceOrder"=0, "sxFieldId"="X_Span", "sxSequenceId"="", "sDisplayName"="X Span", "sValue"="0", "sUnits"="MHz", "nDataType"=enum."numeric", "nNextItem"=enum."Reset", "fSystem"=TRUE, "fSystemValue"=TRUE, "fRequired"=TRUE, "fSetAtTest"=TRUE, "fTestField"=TRUE, "fDeleted"=FALSE, "fIndexed"=FALSE, "fFreeList"=FALSE}, {"ixField"=0, "iSequenceOrder"=0, "sxFieldId"="Y_Max_1", "sxSequenceId"="", "sDisplayName"="Y Max 1", "sValue"="0", "sUnits"="dBm", "nDataType"=enum."numeric", "nNextItem"=enum."Reset", "fSystem"=TRUE, "fSystemValue"=TRUE, "fRequired"=TRUE, "fSetAtTest"=TRUE, "fTestField"=TRUE, "fDeleted"=FALSE, "fIndexed"=FALSE, "fFreeList"=FALSE}, {"ixField"=0, "iSequenceOrder"=0, "sxFieldId"="Y_Max_2", "sxSequenceId"="", "sDisplayName"="Y Max 2", "sValue"="0", "sUnits"="dBc", "nDataType"=enum."numeric", "nNextItem"=enum."Reset", "fSystem"=TRUE, "fSystemValue"=TRUE, "fRequired"=TRUE, "fSetAtTest"=TRUE, "fTestField"=TRUE, "fDeleted"=FALSE, "fIndexed"=FALSE, "fFreeList"=FALSE}, {"ixField"=0, "iSequenceOrder"=0, "sxFieldId"="Y_Min_1", "sxSequenceId"="", "sDisplayName"="Y Min 1", "sValue"="0", "sUnits"="dBm", "nDataType"=enum."numeric", "nNextItem"=enum."Reset", "fSystem"=TRUE, "fSystemValue"=TRUE, "fRequired"=TRUE, "fSetAtTest"=TRUE, "fTestField"=TRUE, "fDeleted"=FALSE, "fIndexed"=FALSE, "fFreeList"=FALSE}, {"ixField"=0, "iSequenceOrder"=0, "sxFieldId"="Y_Min_2", "sxSequenceId"="", "sDisplayName"="Y Min 2", "sValue"="0", "sUnits"="dBc", "nDataType"=enum."numeric", "nNextItem"=enum."Reset", "fSystem"=TRUE, "fSystemValue"=TRUE, "fRequired"=TRUE, "fSetAtTest"=TRUE, "fTestField"=TRUE, "fDeleted"=FALSE, "fIndexed"=FALSE, "fFreeList"=FALSE}, {"ixField"=0, "iSequenceOrder"=0, "sxFieldId"="Limit_Percentage", "sxSequenceId"="", "sDisplayName"="Limit Percentage", "sValue"="100", "sUnits"="%", "nDataType"=enum."numeric", "nNextItem"=enum."Reset", "fSystem"=TRUE, "fSystemValue"=TRUE, "fRequired"=TRUE, "fSetAtTest"=TRUE, "fTestField"=TRUE, "fDeleted"=FALSE, "fIndexed"=FALSE, "fFreeList"=FALSE}]
  in  "QuickMode":i32
  in  "DriverTypes":string[](array[string])=["PIM"]
  in  "Description":string="This test will perform Passive Intermodulation testing using a Passive Intermodulation (PIM) analyzer."
  in  "Version":T4={"Version"="6.3", "Build Number"=12, "Build Date/Time"=3440694548.419435} {"Build Date/Time" format="%<%X\n%x>T"}
  # "Note: The version\nglobal is set during\nbuild.  Don't change\nor rename this variable"
  # "This is an array of fields\nto be added to the DB if\nthis test is placed into a\ntest sequence."
  # "Add a description for this\ntest before building"
  # "Add a list of driver types\n(e.g., PIM,...) required\nby the test (can be empty)"
  # "QuickMode:\n0 = Supported (OFF By Default)\n1 = Supported (ON By Default)\n2 = Not Supported"
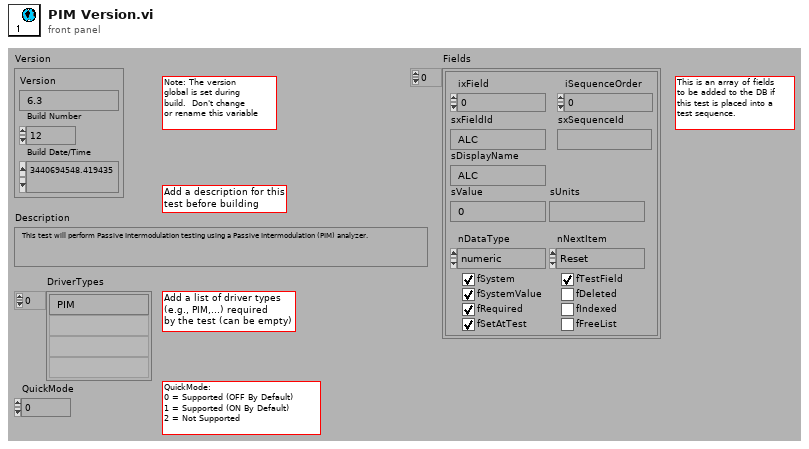
[diagram p1: front panel]
types:
  T1 = typedef "Field Record.ctl" = cluster{"ixField":i32, "iSequenceOrder":i32, "sxFieldId":string, "sxSequenceId":string, "sDisplayName":string, "sValue":string, "sUnits":string, "nDataType":T2, "nNextItem":T3, "fSystem":bool, "fSystemValue":bool, "fRequired":bool, "fSetAtTest":bool, "fTestField":bool, "fDeleted":bool, "fIndexed":bool, "fFreeList":bool}
  T2 = typedef "Field DataTypes.ctl" = enum32{"text", "numeric", "list", "timestamp", "boolean"}
  T3 = typedef "Field NextItem.ctl" = enum32{"Reset", "Retain", "Auto-Increment"}
  T4 = typedef "OGAB Version.ctl" = cluster{"Version":string, "Build Number":u32, "Build Date/Time":dbl}
diagram:
